vi "Read Tiff File (Bitmiracle libtiff.net).vi"(8 "error in (no error)":errorcluster, 11 "Input path":path=path "C:/0_DLPGUI_V2/lowResTest.tif") -> (0 "error out":errorcluster, 2 "ImageData":T1, 3 "Grayscale (U16) Image Data":u16[][][](array[numeric]), 4 "number of frames":i32)   [LabVIEW 2022 SP3]
doc: "This SubVI is a modified version of the file Read Tiff File.vi that is included in the libtiff2.llb library. The libtiff2.llb was provided by Nico_MPI on the NI LabVIEW discussion forum at http://forums.ni.com/t5/LabVIEW/Labview-libtiff-implementation/td-p/929843/page/2.\n\nRead a multipage TIFF returning an array of images and the total number of frames. This VI closes the file after returning the images array."
uses:
  Classes/TopLevel/Typedefs/TiffImageData--Cluster.ctl
  <vilib>/LVH/i3 JSON/JSON Parsing/Get Object Parameter Files/Get Object Parameter - Object.vi
  <vilib>/LVH/i3 JSON/JSON Parsing/Get Array Value at Index Files/Get Array Value at Index - Array.vi
  C:/Nuget/BitMiracle.LibTiff.NET.2.4.649/lib/net40/BitMiracle.LibTiff.NET.dll
  Nuget/BitMiracle.LibTiff.NET.2.4.649/lib/net40/BitMiracle.LibTiff.NET.dll
  BitMiracle.LibTiff.NET.dll
  <vilib>/LVH/i3 JSON/i3-json.lvlib
panel:
  out "Numeric":i32
  out "ImageBufferMain":u8[][](array[numeric])
  out "ChannelTargetMaterials":string[](array[string])
  out "MaterialNames":string[](array[string])
  out "error out 2":errorcluster
  out "Subject":string
  out "0 6":T2(plugin-control)
  out "0 5":T2(plugin-control)
  out "0 4":T2(plugin-control)
  out "0 3":T2(plugin-control)
  out "0 2":T2(plugin-control)
  out "ScanLineSize":i32
  out "0":T2(plugin-control)
  out "element 2":i32
  out "unsigned 8bit integer":u8[][](array[numeric])
  out "buffer":u8[][](array[numeric])
  out "Array":u64[](array[numeric])
  out "element":i32
  out "NumberOfTiles":i32
  out "Number Bytes read 2":i32
  out "Number Bytes read":i32
  out "Grayscale (SGL) Image Data":sgl[][][](array[numeric])
  # "278x1271"
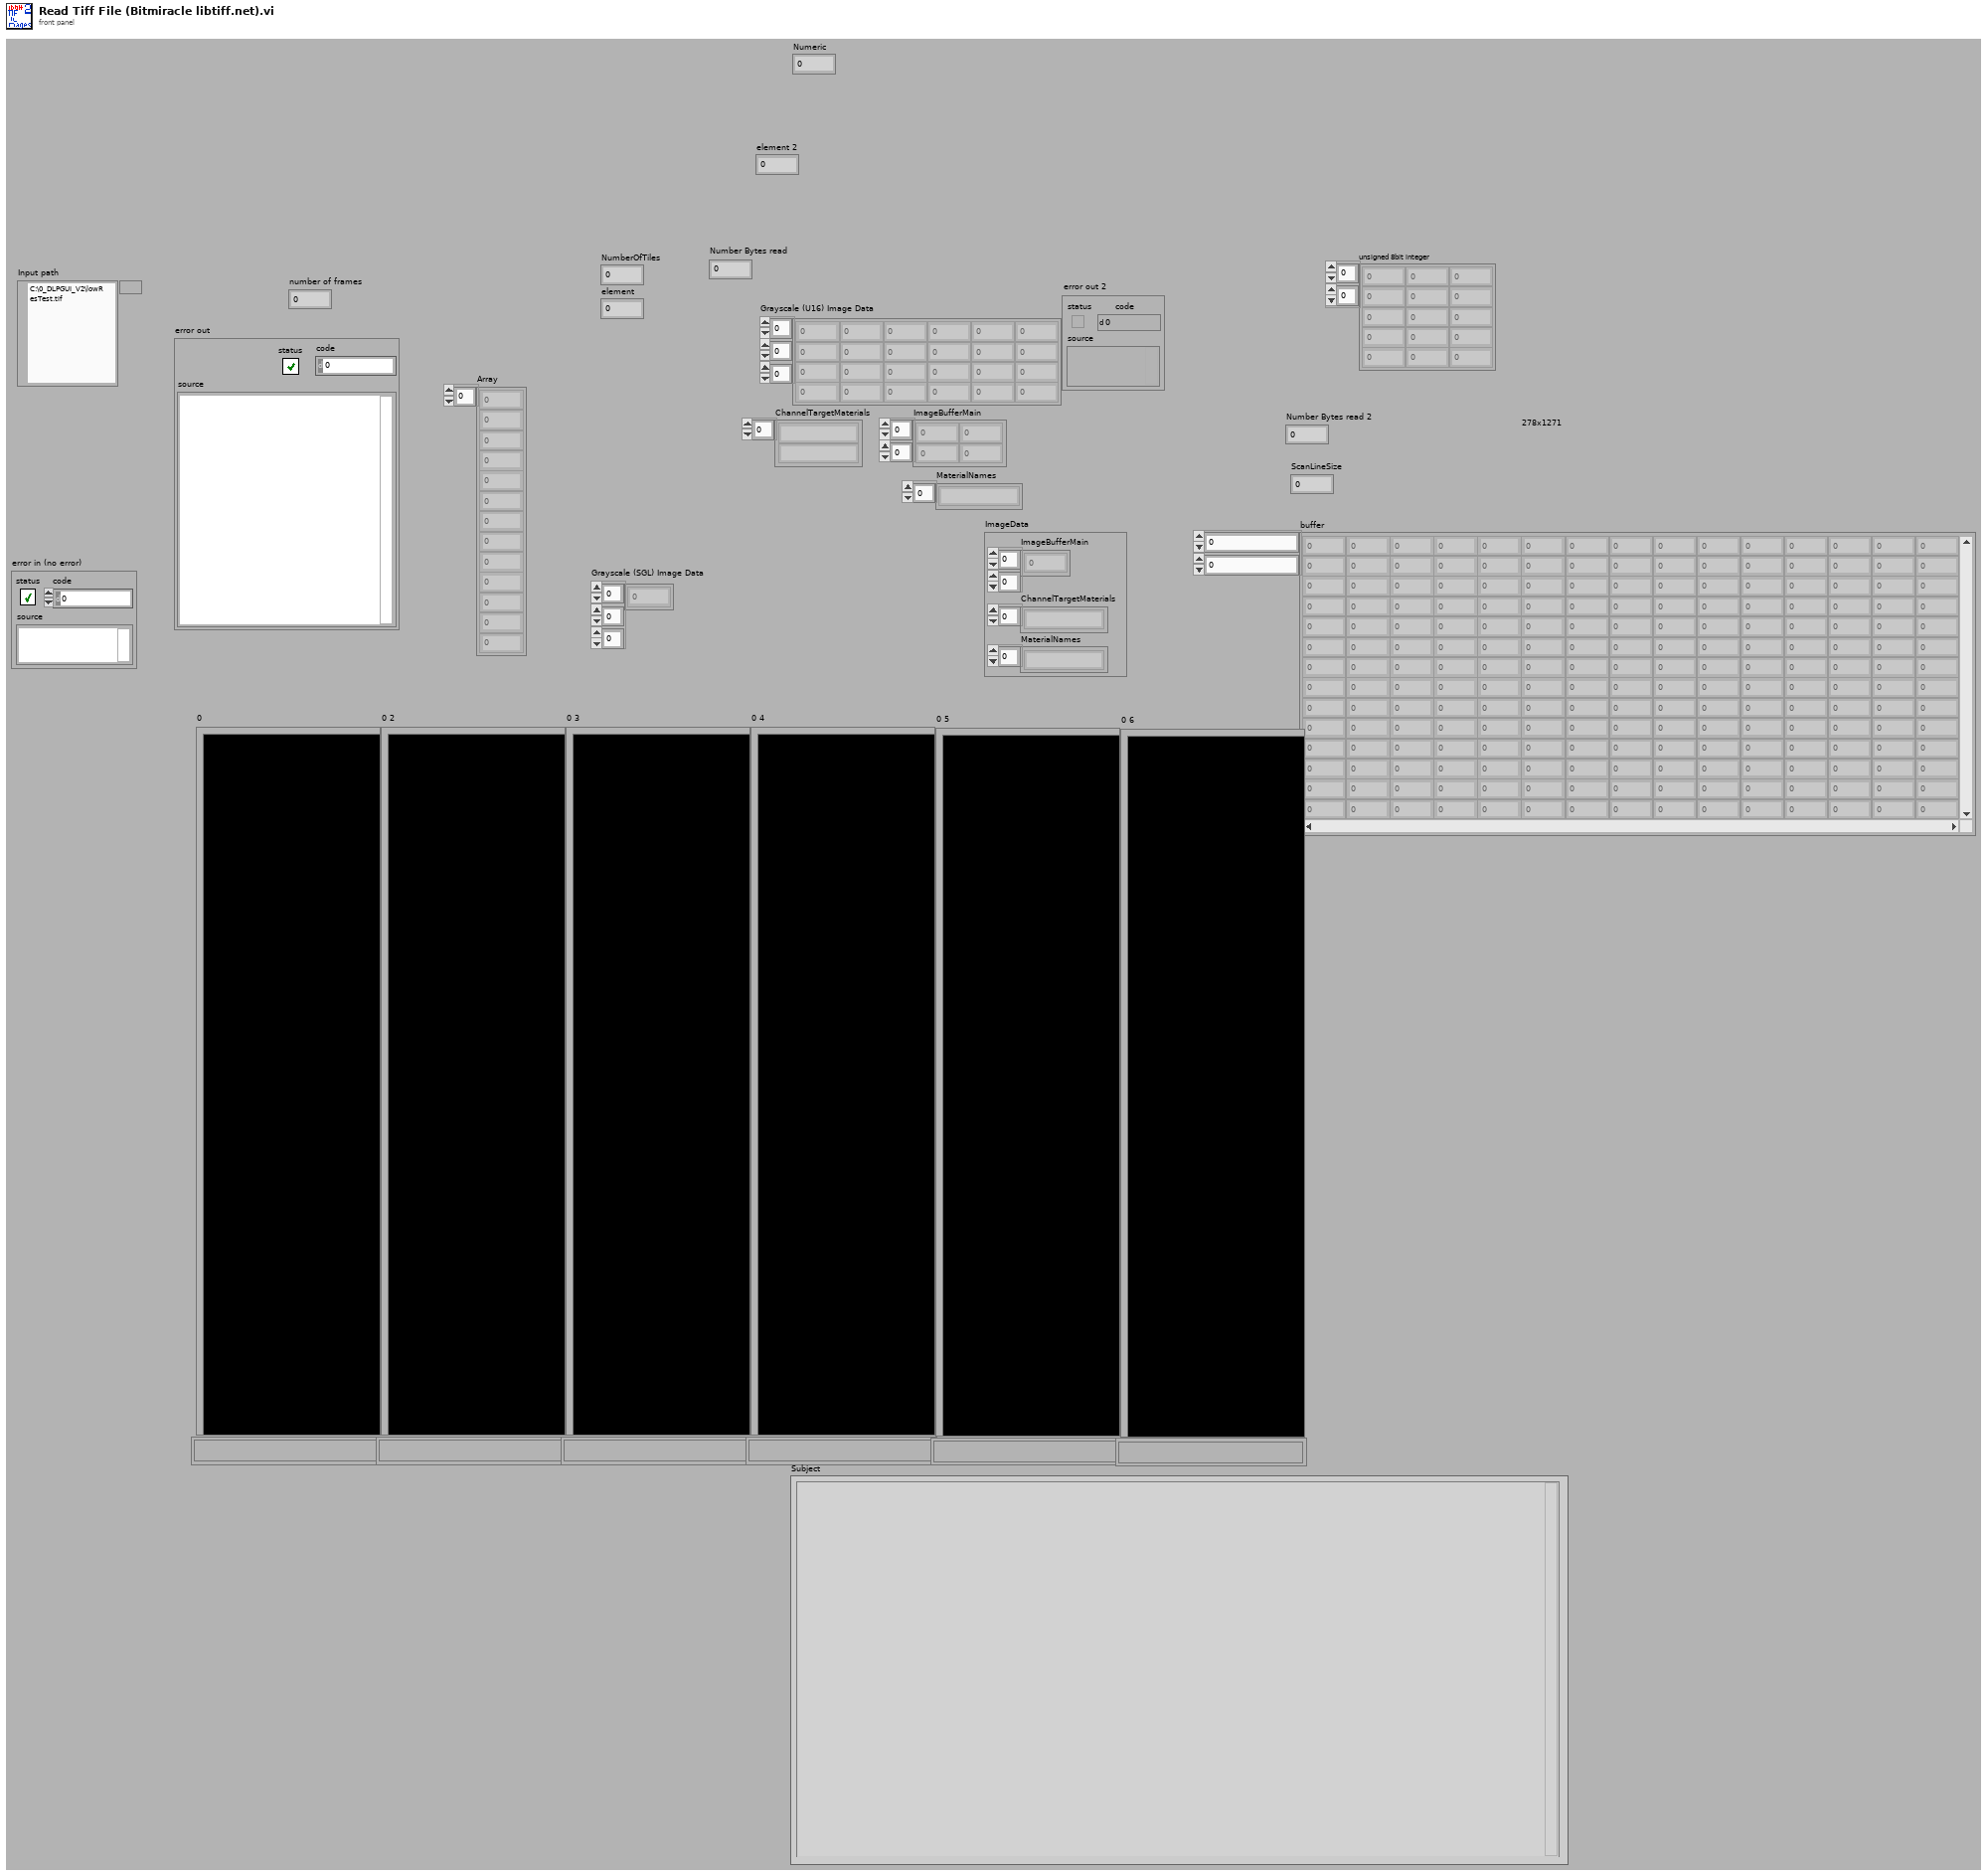
[diagram p1: front panel]
types:
  T1 = typedef "TiffImageData--Cluster.ctl" = cluster{"ImageBufferMain":u8[][], "ChannelTargetMaterials":string[], "MaterialNames":string[]}
  T2 = typedef "IMAQ Image.ctl" = refnum<image>
  T3 = typedef "Image Type" = u32
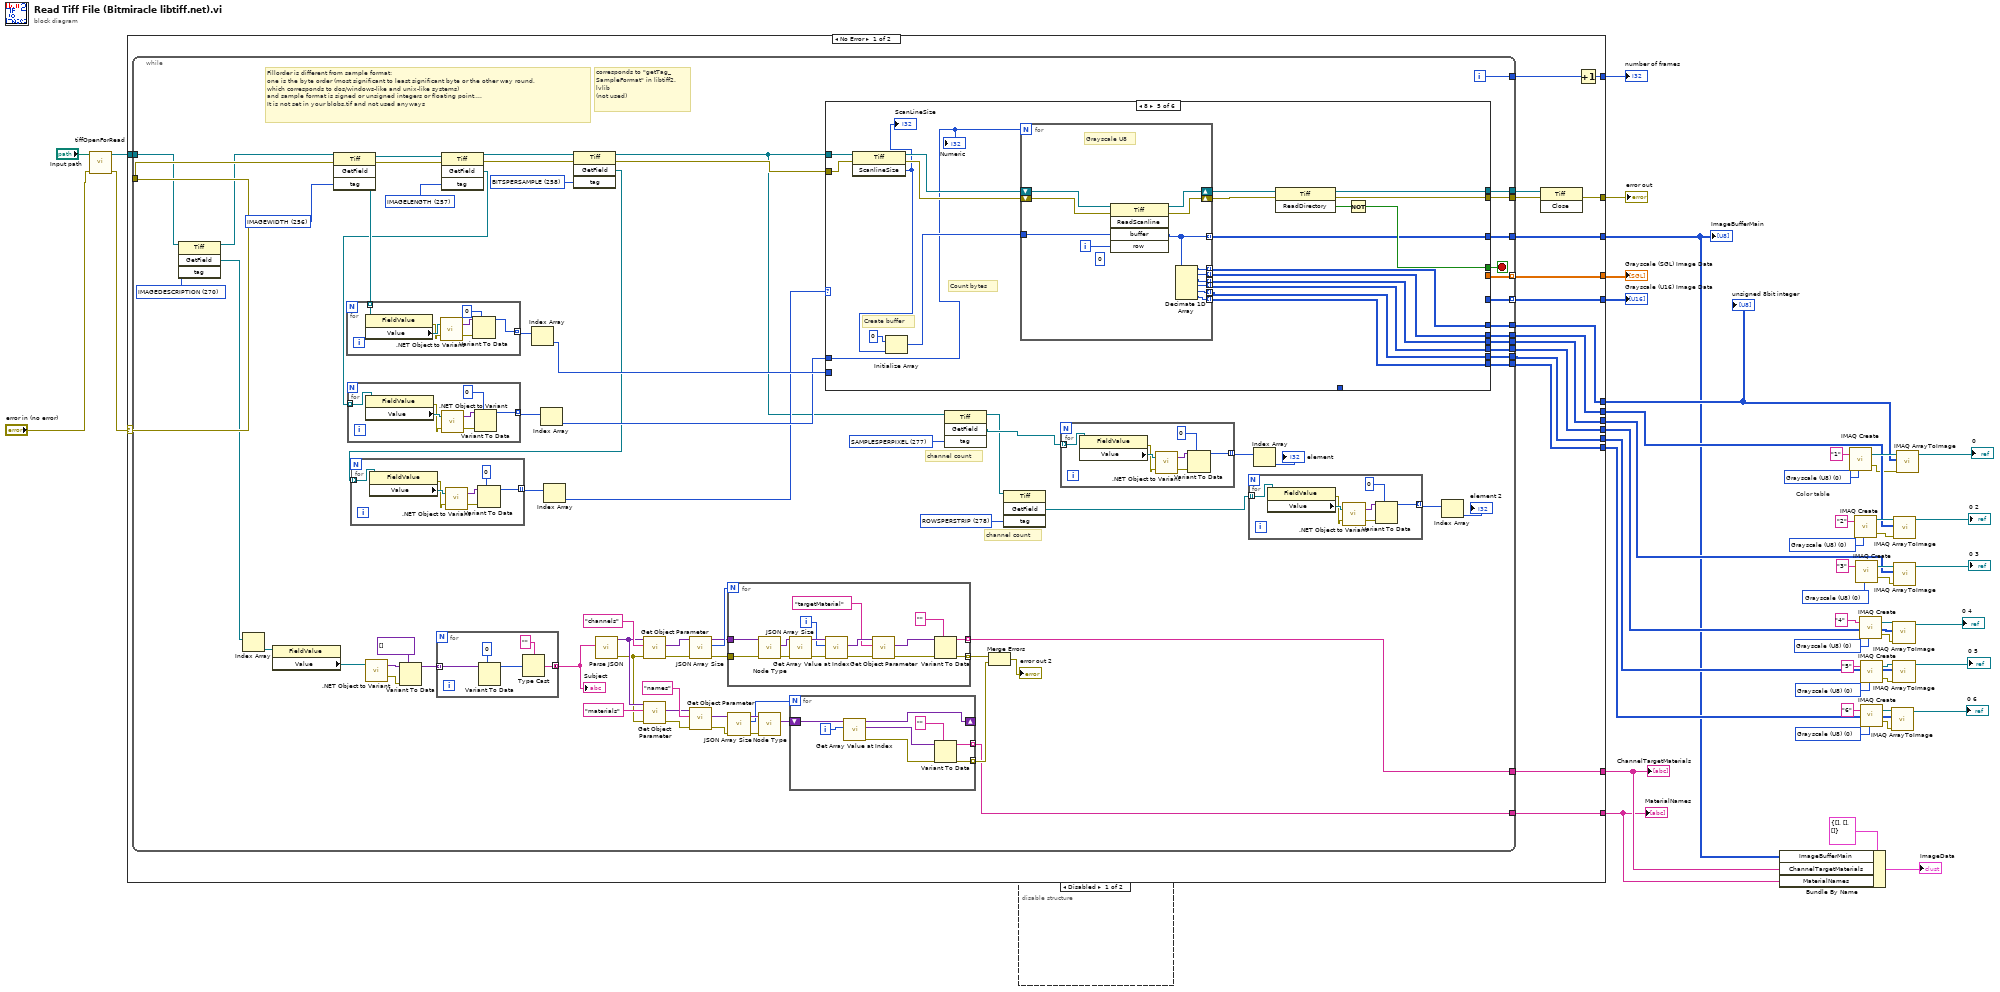
[diagram p0: block diagram]
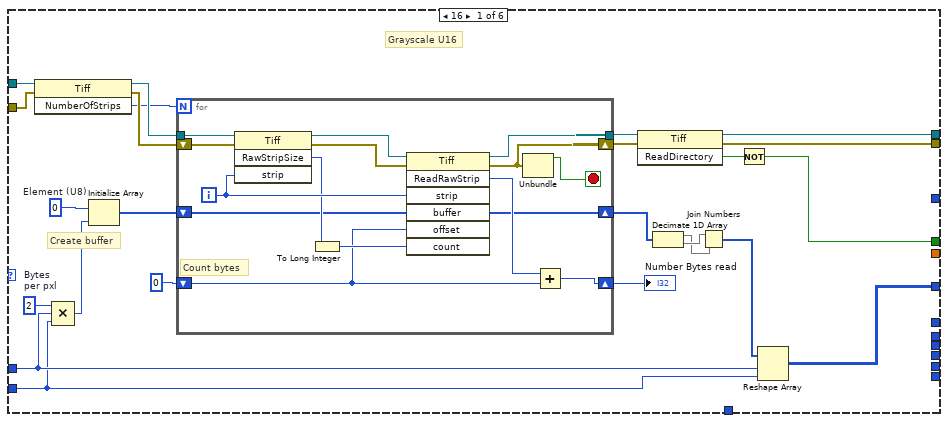
[diagram p3: hidden frame]
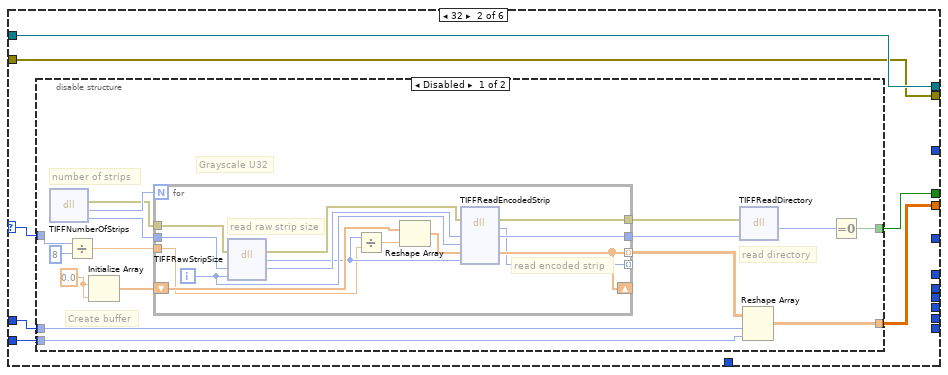
[diagram p4: hidden frame]
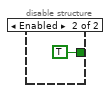
[diagram p5: hidden frame]
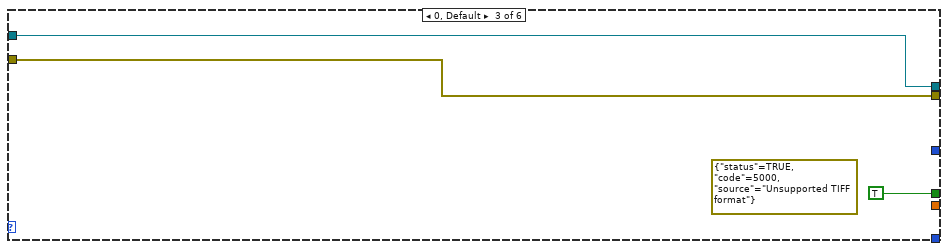
[diagram p6: hidden frame]
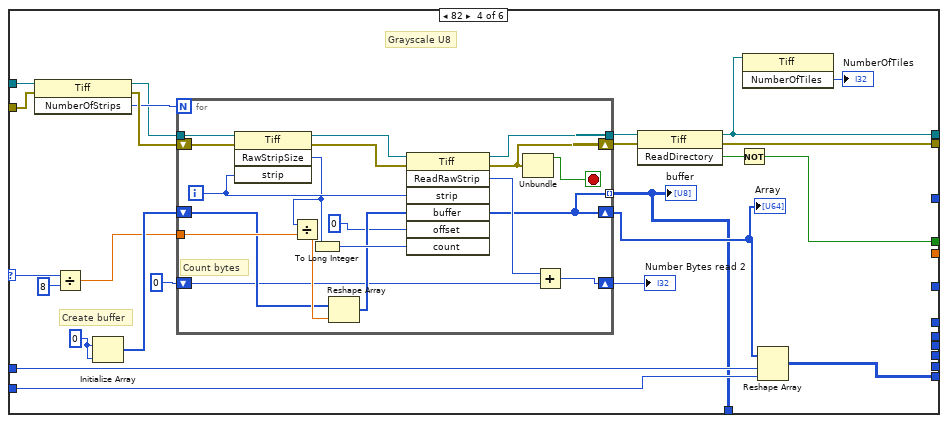
[diagram p7: hidden frame]
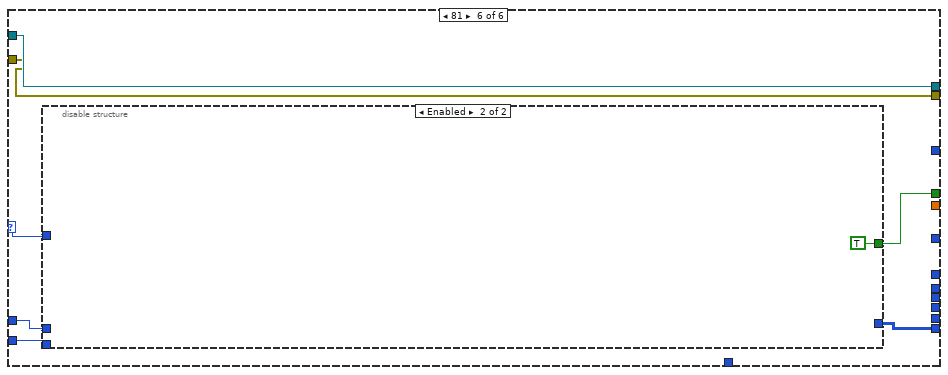
[diagram p8: hidden frame]
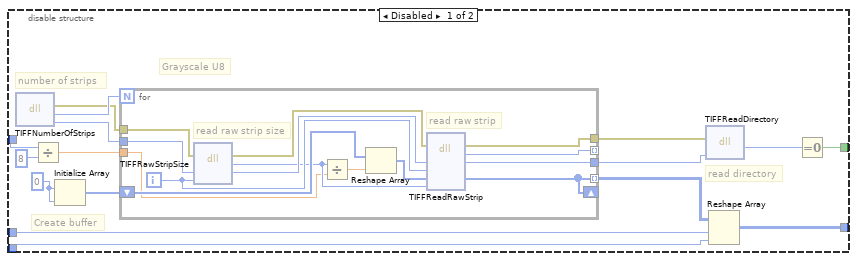
[diagram p9: hidden frame]
diagram:
  w27 = T3 0 items=["Grayscale (U8)", "Grayscale (I16)", "Grayscale (SGL)", "Complex (CSG)", "RGB (U32)", "HSL (U32)", "RGB (U64)", "Grayscale (U16)"] ("Image Type")
  w32 = T3 0 items=["Grayscale (U8)", "Grayscale (I16)", "Grayscale (SGL)", "Complex (CSG)", "RGB (U32)", "HSL (U32)", "RGB (U64)", "Grayscale (U16)"] ("Image Type")
  w29 = T3 0 items=["Grayscale (U8)", "Grayscale (I16)", "Grayscale (SGL)", "Complex (CSG)", "RGB (U32)", "HSL (U32)", "RGB (U64)", "Grayscale (U16)"] ("Image Type")
  w33 = T3 0 items=["Grayscale (U8)", "Grayscale (I16)", "Grayscale (SGL)", "Complex (CSG)", "RGB (U32)", "HSL (U32)", "RGB (U64)", "Grayscale (U16)"] ("Image Type")
  w36 = T3 0 items=["Grayscale (U8)", "Grayscale (I16)", "Grayscale (SGL)", "Complex (CSG)", "RGB (U32)", "HSL (U32)", "RGB (U64)", "Grayscale (U16)"] ("Image Type")
  w40 = T3 0 items=["Grayscale (U8)", "Grayscale (I16)", "Grayscale (SGL)", "Complex (CSG)", "RGB (U32)", "HSL (U32)", "RGB (U64)", "Grayscale (U16)"] ("Image Type")
  # "Color table"
  n1 = call "tiffOpenForRead.vi"("error in (no error)"="error in (no error)", "Path"="Input path") -> ("error out"=w42:errorcluster, "BitMiracle.LibTiff.Classic.Tiff"=w45:refnum<k24>)  [unwired: 8 in]
  n2 = case shown="No Error" w42 {
    selector: w42 -> [w67 w401]
    tunnel: [w65 _] -> w49
    tunnel: [w59 w401] -> w48
    tunnel: [w64 _] -> w47
    tunnel: [w63 _] -> w44
    tunnel: w45 -> [w62 _]
    tunnel: [w58 _] -> w37
    tunnel: [w57 _] -> w24
    tunnel: [w56 _] -> w9
    tunnel: [w55 _] -> w8
    tunnel: [w54 _] -> w7
    tunnel: [w53 _] -> w6
    tunnel: [w52 _] -> w3
    tunnel: [w51 _] -> w2
    tunnel: [w50 _] -> w1
    frame No Error {
      n3 = while {
        tunnel: [w141] -> w66
        tunnel: w67 -> [w102]
        tunnel: [w137] -> w63 mode=indexing
        tunnel: [w140] -> w64 mode=indexing
        tunnel: w62 -> [w101]
        tunnel: [w139] -> w61
        tunnel: [w138] -> w60
        tunnel: [w114] -> w53
        tunnel: [w108] -> w58
        tunnel: [w107] -> w57
        tunnel: [w106] -> w56
        tunnel: [w105] -> w55
        tunnel: [w104] -> w54
        tunnel: [w70] -> w52
        tunnel: [w69] -> w51
        tunnel: [w68] -> w50
        i -> [w141]
        stop <- w142 stop-if-true
        w103 = 270 items=["IGNORE"=0, "SUBFILETYPE"=254, "OSUBFILETYPE"=255, "IMAGEWIDTH"=256, "IMAGELENGTH"=257, "BITSPERSAMPLE"=258, "COMPRESSION"=259, "PHOTOMETRIC"=262, "THRESHHOLDING"=263, "CELLWIDTH"=264, "CELLLENGTH"=265, "FILLORDER"=266, "DOCUMENTNAME"=269, "IMAGEDESCRIPTION"=270, "MAKE"=271, "MODEL"=272, "STRIPOFFSETS"=273, "ORIENTATION"=274, "SAMPLESPERPIXEL"=277, "ROWSPERSTRIP"=278, "STRIPBYTECOUNTS"=279, "MINSAMPLEVALUE"=280, "MAXSAMPLEVALUE"=281, "XRESOLUTION"=282, "YRESOLUTION"=283, "PLANARCONFIG"=284, "PAGENAME"=285, "XPOSITION"=286, "YPOSITION"=287, "FREEOFFSETS"=288, "FREEBYTECOUNTS"=289, "GRAYRESPONSEUNIT"=290, "GRAYRESPONSECURVE"=291, "GROUP3OPTIONS, T4OPTIONS"=292, "GROUP4OPTIONS, T6OPTIONS"=293, "RESOLUTIONUNIT"=296, "PAGENUMBER"=297, "COLORRESPONSEUNIT"=300, "TRANSFERFUNCTION"=301, "SOFTWARE"=305, "DATETIME"=306, "ARTIST"=315, "HOSTCOMPUTER"=316, "PREDICTOR"=317, "WHITEPOINT"=318, "PRIMARYCHROMATICITIES"=319, "COLORMAP"=320, "HALFTONEHINTS"=321, "TILEWIDTH"=322, "TILELENGTH"=323, "TILEOFFSETS"=324, "TILEBYTECOUNTS"=325, "BADFAXLINES"=326, "CLEANFAXDATA"=327, "CONSECUTIVEBADFAXLINES"=328, "SUBIFD"=330, "INKSET"=332, "INKNAMES"=333, "NUMBEROFINKS"=334, "DOTRANGE"=336, "TARGETPRINTER"=337, "EXTRASAMPLES"=338, "SAMPLEFORMAT"=339, "SMINSAMPLEVALUE"=340, "SMAXSAMPLEVALUE"=341, "CLIPPATH"=343, "XCLIPPATHUNITS"=344, "YCLIPPATHUNITS"=345, "INDEXED"=346, "JPEGTABLES"=347, "OPIPROXY"=351, "JPEGPROC"=512, "JPEGIFOFFSET"=513, "JPEGIFBYTECOUNT"=514, "JPEGRESTARTINTERVAL"=515, "JPEGLOSSLESSPREDICTORS"=517, "JPEGPOINTTRANSFORM"=518, "JPEGQTABLES"=519, "JPEGDCTABLES"=520, "JPEGACTABLES"=521, "YCBCRCOEFFICIENTS"=529, "YCBCRSUBSAMPLING"=530, "YCBCRPOSITIONING"=531, "REFERENCEBLACKWHITE"=532, "XMLPACKET"=700, "OPIIMAGEID"=32781, "REFPTS"=32953, "REGIONTACKPOINT"=32954, "REGIONWARPCORNERS"=32955, "REGIONAFFINE"=32956, "MATTEING"=32995, "DATATYPE"=32996, "IMAGEDEPTH"=32997, "TILEDEPTH"=32998, "PIXAR_IMAGEFULLWIDTH"=33300, "PIXAR_IMAGEFULLLENGTH"=33301, "PIXAR_TEXTUREFORMAT"=33302, "PIXAR_WRAPMODES"=33303, "PIXAR_FOVCOT"=33304, "PIXAR_MATRIX_WORLDTOSCREEN"=33305, "PIXAR_MATRIX_WORLDTOCAMERA"=33306, "WRITERSERIALNUMBER"=33405, "COPYRIGHT"=33432, "EXIF_EXPOSURETIME"=33434, "EXIF_FNUMBER"=33437, "GEOTIFF_MODELPIXELSCALETAG"=33550, "RICHTIFFIPTC"=33723, "GEOTIFF_MODELTIEPOINTTAG"=33922, "IT8SITE"=34016, "IT8COLORSEQUENCE"=34017, "IT8HEADER"=34018, "IT8RASTERPADDING"=34019, "IT8BITSPERRUNLENGTH"=34020, "IT8BITSPEREXTENDEDRUNLENGTH"=34021, "IT8COLORTABLE"=34022, "IT8IMAGECOLORINDICATOR"=34023, "IT8BKGCOLORINDICATOR"=34024, "IT8IMAGECOLORVALUE"=34025, "IT8BKGCOLORVALUE"=34026, "IT8PIXELINTENSITYRANGE"=34027, "IT8TRANSPARENCYINDICATOR"=34028, "IT8COLORCHARACTERIZATION"=34029, "IT8HCUSAGE"=34030, "IT8TRAPINDICATOR"=34031, "IT8CMYKEQUIVALENT"=34032, "FRAMECOUNT"=34232, "GEOTIFF_MODELTRANSFORMATIONTAG"=34264, "PHOTOSHOP"=34377, "EXIFIFD"=34665, "ICCPROFILE"=34675, "GEOTIFF_GEOKEYDIRECTORYTAG"=34735, "GEOTIFF_GEODOUBLEPARAMSTAG"=34736, "GEOTIFF_GEOASCIIPARAMSTAG"=34737, "JBIGOPTIONS"=34750, "EXIF_EXPOSUREPROGRAM"=34850, "EXIF_SPECTRALSENSITIVITY"=34852, "GPSIFD"=34853, "EXIF_ISOSPEEDRATINGS"=34855, "EXIF_OECF"=34856, "FAXRECVPARAMS"=34908, "FAXSUBADDRESS"=34909, "FAXRECVTIME"=34910, "FAXDCS"=34911, "FEDEX_EDR"=34929, "EXIF_EXIFVERSION"=36864, "EXIF_DATETIMEORIGINAL"=36867, "EXIF_DATETIMEDIGITIZED"=36868, "EXIF_COMPONENTSCONFIGURATION"=37121, "EXIF_COMPRESSEDBITSPERPIXEL"=37122, "EXIF_SHUTTERSPEEDVALUE"=37377, "EXIF_APERTUREVALUE"=37378, "EXIF_BRIGHTNESSVALUE"=37379, "EXIF_EXPOSUREBIASVALUE"=37380, "EXIF_MAXAPERTUREVALUE"=37381, "EXIF_SUBJECTDISTANCE"=37382, "EXIF_METERINGMODE"=37383, "EXIF_LIGHTSOURCE"=37384, "EXIF_FLASH"=37385, "EXIF_FOCALLENGTH"=37386, "EXIF_SUBJECTAREA"=37396, "STONITS"=37439, "EXIF_MAKERNOTE"=37500, "EXIF_USERCOMMENT"=37510, "EXIF_SUBSECTIME"=37520, "EXIF_SUBSECTIMEORIGINAL"=37521, "EXIF_SUBSECTIMEDIGITIZED"=37522, "EXIF_FLASHPIXVERSION"=40960, "EXIF_COLORSPACE"=40961, "EXIF_PIXELXDIMENSION"=40962, "EXIF_PIXELYDIMENSION"=40963, "EXIF_RELATEDSOUNDFILE"=40964, "INTEROPERABILITYIFD"=40965, "EXIF_FLASHENERGY"=41483, "EXIF_SPATIALFREQUENCYRESPONSE"=41484, "EXIF_FOCALPLANEXRESOLUTION"=41486, "EXIF_FOCALPLANEYRESOLUTION"=41487, "EXIF_FOCALPLANERESOLUTIONUNIT"=41488, "EXIF_SUBJECTLOCATION"=41492, "EXIF_EXPOSUREINDEX"=41493, "EXIF_SENSINGMETHOD"=41495, "EXIF_FILESOURCE"=41728, "EXIF_SCENETYPE"=41729, "EXIF_CFAPATTERN"=41730, "EXIF_CUSTOMRENDERED"=41985, "EXIF_EXPOSUREMODE"=41986, "EXIF_WHITEBALANCE"=41987, "EXIF_DIGITALZOOMRATIO"=41988, "EXIF_FOCALLENGTHIN35MMFILM"=41989, "EXIF_SCENECAPTURETYPE"=41990, "EXIF_GAINCONTROL"=41991, "EXIF_CONTRAST"=41992, "EXIF_SATURATION"=41993, "EXIF_SHARPNESS"=41994, "EXIF_DEVICESETTINGDESCRIPTION"=41995, "EXIF_SUBJECTDISTANCERANGE"=41996, "EXIF_IMAGEUNIQUEID"=42016, "DNGVERSION"=50706, "DNGBACKWARDVERSION"=50707, "UNIQUECAMERAMODEL"=50708, "LOCALIZEDCAMERAMODEL"=50709, "CFAPLANECOLOR"=50710, "CFALAYOUT"=50711, "LINEARIZATIONTABLE"=50712, "BLACKLEVELREPEATDIM"=50713, "BLACKLEVEL"=50714, "BLACKLEVELDELTAH"=50715, "BLACKLEVELDELTAV"=50716, "WHITELEVEL"=50717, "DEFAULTSCALE"=50718, "DEFAULTCROPORIGIN"=50719, "DEFAULTCROPSIZE"=50720, "COLORMATRIX1"=50721, "COLORMATRIX2"=50722, "CAMERACALIBRATION1"=50723, "CAMERACALIBRATION2"=50724, "REDUCTIONMATRIX1"=50725, "REDUCTIONMATRIX2"=50726, "ANALOGBALANCE"=50727, "ASSHOTNEUTRAL"=50728, "ASSHOTWHITEXY"=50729, "BASELINEEXPOSURE"=50730, "BASELINENOISE"=50731, "BASELINESHARPNESS"=50732, "BAYERGREENSPLIT"=50733, "LINEARRESPONSELIMIT"=50734, "CAMERASERIALNUMBER"=50735, "LENSINFO"=50736, "CHROMABLURRADIUS"=50737, "ANTIALIASSTRENGTH"=50738, "SHADOWSCALE"=50739, "DNGPRIVATEDATA"=50740, "MAKERNOTESAFETY"=50741, "CALIBRATIONILLUMINANT1"=50778, "CALIBRATIONILLUMINANT2"=50779, "BESTQUALITYSCALE"=50780, "RAWDATAUNIQUEID"=50781, "ORIGINALRAWFILENAME"=50827, "ORIGINALRAWFILEDATA"=50828, "ACTIVEAREA"=50829, "MASKEDAREAS"=50830, "ASSHOTICCPROFILE"=50831, "ASSHOTPREPROFILEMATRIX"=50832, "CURRENTICCPROFILE"=50833, "CURRENTPREPROFILEMATRIX"=50834, "DCSHUESHIFTVALUES"=65535, "FAXMODE"=65536, "JPEGQUALITY"=65537, "JPEGCOLORMODE"=65538, "JPEGTABLESMODE"=65539, "FAXFILLFUNC"=65540, "PIXARLOGDATAFMT"=65549, "DCSIMAGERTYPE"=65550, "DCSINTERPMODE"=65551, "DCSBALANCEARRAY"=65552, "DCSCORRECTMATRIX"=65553, "DCSGAMMA"=65554, "DCSTOESHOULDERPTS"=65555, "DCSCALIBRATIONFD"=65556, "ZIPQUALITY"=65557, "PIXARLOGQUALITY"=65558, "DCSCLIPRECTANGLE"=65559, "SGILOGDATAFMT"=65560, "SGILOGENCODE"=65561] ("tag")
        w113 = 278 items=["IGNORE"=0, "SUBFILETYPE"=254, "OSUBFILETYPE"=255, "IMAGEWIDTH"=256, "IMAGELENGTH"=257, "BITSPERSAMPLE"=258, "COMPRESSION"=259, "PHOTOMETRIC"=262, "THRESHHOLDING"=263, "CELLWIDTH"=264, "CELLLENGTH"=265, "FILLORDER"=266, "DOCUMENTNAME"=269, "IMAGEDESCRIPTION"=270, "MAKE"=271, "MODEL"=272, "STRIPOFFSETS"=273, "ORIENTATION"=274, "SAMPLESPERPIXEL"=277, "ROWSPERSTRIP"=278, "STRIPBYTECOUNTS"=279, "MINSAMPLEVALUE"=280, "MAXSAMPLEVALUE"=281, "XRESOLUTION"=282, "YRESOLUTION"=283, "PLANARCONFIG"=284, "PAGENAME"=285, "XPOSITION"=286, "YPOSITION"=287, "FREEOFFSETS"=288, "FREEBYTECOUNTS"=289, "GRAYRESPONSEUNIT"=290, "GRAYRESPONSECURVE"=291, "GROUP3OPTIONS, T4OPTIONS"=292, "GROUP4OPTIONS, T6OPTIONS"=293, "RESOLUTIONUNIT"=296, "PAGENUMBER"=297, "COLORRESPONSEUNIT"=300, "TRANSFERFUNCTION"=301, "SOFTWARE"=305, "DATETIME"=306, "ARTIST"=315, "HOSTCOMPUTER"=316, "PREDICTOR"=317, "WHITEPOINT"=318, "PRIMARYCHROMATICITIES"=319, "COLORMAP"=320, "HALFTONEHINTS"=321, "TILEWIDTH"=322, "TILELENGTH"=323, "TILEOFFSETS"=324, "TILEBYTECOUNTS"=325, "BADFAXLINES"=326, "CLEANFAXDATA"=327, "CONSECUTIVEBADFAXLINES"=328, "SUBIFD"=330, "INKSET"=332, "INKNAMES"=333, "NUMBEROFINKS"=334, "DOTRANGE"=336, "TARGETPRINTER"=337, "EXTRASAMPLES"=338, "SAMPLEFORMAT"=339, "SMINSAMPLEVALUE"=340, "SMAXSAMPLEVALUE"=341, "CLIPPATH"=343, "XCLIPPATHUNITS"=344, "YCLIPPATHUNITS"=345, "INDEXED"=346, "JPEGTABLES"=347, "OPIPROXY"=351, "JPEGPROC"=512, "JPEGIFOFFSET"=513, "JPEGIFBYTECOUNT"=514, "JPEGRESTARTINTERVAL"=515, "JPEGLOSSLESSPREDICTORS"=517, "JPEGPOINTTRANSFORM"=518, "JPEGQTABLES"=519, "JPEGDCTABLES"=520, "JPEGACTABLES"=521, "YCBCRCOEFFICIENTS"=529, "YCBCRSUBSAMPLING"=530, "YCBCRPOSITIONING"=531, "REFERENCEBLACKWHITE"=532, "XMLPACKET"=700, "OPIIMAGEID"=32781, "REFPTS"=32953, "REGIONTACKPOINT"=32954, "REGIONWARPCORNERS"=32955, "REGIONAFFINE"=32956, "MATTEING"=32995, "DATATYPE"=32996, "IMAGEDEPTH"=32997, "TILEDEPTH"=32998, "PIXAR_IMAGEFULLWIDTH"=33300, "PIXAR_IMAGEFULLLENGTH"=33301, "PIXAR_TEXTUREFORMAT"=33302, "PIXAR_WRAPMODES"=33303, "PIXAR_FOVCOT"=33304, "PIXAR_MATRIX_WORLDTOSCREEN"=33305, "PIXAR_MATRIX_WORLDTOCAMERA"=33306, "WRITERSERIALNUMBER"=33405, "COPYRIGHT"=33432, "EXIF_EXPOSURETIME"=33434, "EXIF_FNUMBER"=33437, "RICHTIFFIPTC"=33723, "IT8SITE"=34016, "IT8COLORSEQUENCE"=34017, "IT8HEADER"=34018, "IT8RASTERPADDING"=34019, "IT8BITSPERRUNLENGTH"=34020, "IT8BITSPEREXTENDEDRUNLENGTH"=34021, "IT8COLORTABLE"=34022, "IT8IMAGECOLORINDICATOR"=34023, "IT8BKGCOLORINDICATOR"=34024, "IT8IMAGECOLORVALUE"=34025, "IT8BKGCOLORVALUE"=34026, "IT8PIXELINTENSITYRANGE"=34027, "IT8TRANSPARENCYINDICATOR"=34028, "IT8COLORCHARACTERIZATION"=34029, "IT8HCUSAGE"=34030, "IT8TRAPINDICATOR"=34031, "IT8CMYKEQUIVALENT"=34032, "FRAMECOUNT"=34232, "PHOTOSHOP"=34377, "EXIFIFD"=34665, "ICCPROFILE"=34675, "JBIGOPTIONS"=34750, "EXIF_EXPOSUREPROGRAM"=34850, "EXIF_SPECTRALSENSITIVITY"=34852, "GPSIFD"=34853, "EXIF_ISOSPEEDRATINGS"=34855, "EXIF_OECF"=34856, "FAXRECVPARAMS"=34908, "FAXSUBADDRESS"=34909, "FAXRECVTIME"=34910, "FAXDCS"=34911, "FEDEX_EDR"=34929, "EXIF_EXIFVERSION"=36864, "EXIF_DATETIMEORIGINAL"=36867, "EXIF_DATETIMEDIGITIZED"=36868, "EXIF_COMPONENTSCONFIGURATION"=37121, "EXIF_COMPRESSEDBITSPERPIXEL"=37122, "EXIF_SHUTTERSPEEDVALUE"=37377, "EXIF_APERTUREVALUE"=37378, "EXIF_BRIGHTNESSVALUE"=37379, "EXIF_EXPOSUREBIASVALUE"=37380, "EXIF_MAXAPERTUREVALUE"=37381, "EXIF_SUBJECTDISTANCE"=37382, "EXIF_METERINGMODE"=37383, "EXIF_LIGHTSOURCE"=37384, "EXIF_FLASH"=37385, "EXIF_FOCALLENGTH"=37386, "EXIF_SUBJECTAREA"=37396, "STONITS"=37439, "EXIF_MAKERNOTE"=37500, "EXIF_USERCOMMENT"=37510, "EXIF_SUBSECTIME"=37520, "EXIF_SUBSECTIMEORIGINAL"=37521, "EXIF_SUBSECTIMEDIGITIZED"=37522, "EXIF_FLASHPIXVERSION"=40960, "EXIF_COLORSPACE"=40961, "EXIF_PIXELXDIMENSION"=40962, "EXIF_PIXELYDIMENSION"=40963, "EXIF_RELATEDSOUNDFILE"=40964, "INTEROPERABILITYIFD"=40965, "EXIF_FLASHENERGY"=41483, "EXIF_SPATIALFREQUENCYRESPONSE"=41484, "EXIF_FOCALPLANEXRESOLUTION"=41486, "EXIF_FOCALPLANEYRESOLUTION"=41487, "EXIF_FOCALPLANERESOLUTIONUNIT"=41488, "EXIF_SUBJECTLOCATION"=41492, "EXIF_EXPOSUREINDEX"=41493, "EXIF_SENSINGMETHOD"=41495, "EXIF_FILESOURCE"=41728, "EXIF_SCENETYPE"=41729, "EXIF_CFAPATTERN"=41730, "EXIF_CUSTOMRENDERED"=41985, "EXIF_EXPOSUREMODE"=41986, "EXIF_WHITEBALANCE"=41987, "EXIF_DIGITALZOOMRATIO"=41988, "EXIF_FOCALLENGTHIN35MMFILM"=41989, "EXIF_SCENECAPTURETYPE"=41990, "EXIF_GAINCONTROL"=41991, "EXIF_CONTRAST"=41992, "EXIF_SATURATION"=41993, "EXIF_SHARPNESS"=41994, "EXIF_DEVICESETTINGDESCRIPTION"=41995, "EXIF_SUBJECTDISTANCERANGE"=41996, "EXIF_IMAGEUNIQUEID"=42016, "DNGVERSION"=50706, "DNGBACKWARDVERSION"=50707, "UNIQUECAMERAMODEL"=50708, "LOCALIZEDCAMERAMODEL"=50709, "CFAPLANECOLOR"=50710, "CFALAYOUT"=50711, "LINEARIZATIONTABLE"=50712, "BLACKLEVELREPEATDIM"=50713, "BLACKLEVEL"=50714, "BLACKLEVELDELTAH"=50715, "BLACKLEVELDELTAV"=50716, "WHITELEVEL"=50717, "DEFAULTSCALE"=50718, "DEFAULTCROPORIGIN"=50719, "DEFAULTCROPSIZE"=50720, "COLORMATRIX1"=50721, "COLORMATRIX2"=50722, "CAMERACALIBRATION1"=50723, "CAMERACALIBRATION2"=50724, "REDUCTIONMATRIX1"=50725, "REDUCTIONMATRIX2"=50726, "ANALOGBALANCE"=50727, "ASSHOTNEUTRAL"=50728, "ASSHOTWHITEXY"=50729, "BASELINEEXPOSURE"=50730, "BASELINENOISE"=50731, "BASELINESHARPNESS"=50732, "BAYERGREENSPLIT"=50733, "LINEARRESPONSELIMIT"=50734, "CAMERASERIALNUMBER"=50735, "LENSINFO"=50736, "CHROMABLURRADIUS"=50737, "ANTIALIASSTRENGTH"=50738, "SHADOWSCALE"=50739, "DNGPRIVATEDATA"=50740, "MAKERNOTESAFETY"=50741, "CALIBRATIONILLUMINANT1"=50778, "CALIBRATIONILLUMINANT2"=50779, "BESTQUALITYSCALE"=50780, "RAWDATAUNIQUEID"=50781, "ORIGINALRAWFILENAME"=50827, "ORIGINALRAWFILEDATA"=50828, "ACTIVEAREA"=50829, "MASKEDAREAS"=50830, "ASSHOTICCPROFILE"=50831, "ASSHOTPREPROFILEMATRIX"=50832, "CURRENTICCPROFILE"=50833, "CURRENTPREPROFILEMATRIX"=50834, "DCSHUESHIFTVALUES"=65535, "FAXMODE"=65536, "JPEGQUALITY"=65537, "JPEGCOLORMODE"=65538, "JPEGTABLESMODE"=65539, "FAXFILLFUNC"=65540, "PIXARLOGDATAFMT"=65549, "DCSIMAGERTYPE"=65550, "DCSINTERPMODE"=65551, "DCSBALANCEARRAY"=65552, "DCSCORRECTMATRIX"=65553, "DCSGAMMA"=65554, "DCSTOESHOULDERPTS"=65555, "DCSCALIBRATIONFD"=65556, "ZIPQUALITY"=65557, "PIXARLOGQUALITY"=65558, "DCSCLIPRECTANGLE"=65559, "SGILOGDATAFMT"=65560, "SGILOGENCODE"=65561] ("tag")
        w119 = 277 items=["IGNORE"=0, "SUBFILETYPE"=254, "OSUBFILETYPE"=255, "IMAGEWIDTH"=256, "IMAGELENGTH"=257, "BITSPERSAMPLE"=258, "COMPRESSION"=259, "PHOTOMETRIC"=262, "THRESHHOLDING"=263, "CELLWIDTH"=264, "CELLLENGTH"=265, "FILLORDER"=266, "DOCUMENTNAME"=269, "IMAGEDESCRIPTION"=270, "MAKE"=271, "MODEL"=272, "STRIPOFFSETS"=273, "ORIENTATION"=274, "SAMPLESPERPIXEL"=277, "ROWSPERSTRIP"=278, "STRIPBYTECOUNTS"=279, "MINSAMPLEVALUE"=280, "MAXSAMPLEVALUE"=281, "XRESOLUTION"=282, "YRESOLUTION"=283, "PLANARCONFIG"=284, "PAGENAME"=285, "XPOSITION"=286, "YPOSITION"=287, "FREEOFFSETS"=288, "FREEBYTECOUNTS"=289, "GRAYRESPONSEUNIT"=290, "GRAYRESPONSECURVE"=291, "GROUP3OPTIONS, T4OPTIONS"=292, "GROUP4OPTIONS, T6OPTIONS"=293, "RESOLUTIONUNIT"=296, "PAGENUMBER"=297, "COLORRESPONSEUNIT"=300, "TRANSFERFUNCTION"=301, "SOFTWARE"=305, "DATETIME"=306, "ARTIST"=315, "HOSTCOMPUTER"=316, "PREDICTOR"=317, "WHITEPOINT"=318, "PRIMARYCHROMATICITIES"=319, "COLORMAP"=320, "HALFTONEHINTS"=321, "TILEWIDTH"=322, "TILELENGTH"=323, "TILEOFFSETS"=324, "TILEBYTECOUNTS"=325, "BADFAXLINES"=326, "CLEANFAXDATA"=327, "CONSECUTIVEBADFAXLINES"=328, "SUBIFD"=330, "INKSET"=332, "INKNAMES"=333, "NUMBEROFINKS"=334, "DOTRANGE"=336, "TARGETPRINTER"=337, "EXTRASAMPLES"=338, "SAMPLEFORMAT"=339, "SMINSAMPLEVALUE"=340, "SMAXSAMPLEVALUE"=341, "CLIPPATH"=343, "XCLIPPATHUNITS"=344, "YCLIPPATHUNITS"=345, "INDEXED"=346, "JPEGTABLES"=347, "OPIPROXY"=351, "JPEGPROC"=512, "JPEGIFOFFSET"=513, "JPEGIFBYTECOUNT"=514, "JPEGRESTARTINTERVAL"=515, "JPEGLOSSLESSPREDICTORS"=517, "JPEGPOINTTRANSFORM"=518, "JPEGQTABLES"=519, "JPEGDCTABLES"=520, "JPEGACTABLES"=521, "YCBCRCOEFFICIENTS"=529, "YCBCRSUBSAMPLING"=530, "YCBCRPOSITIONING"=531, "REFERENCEBLACKWHITE"=532, "XMLPACKET"=700, "OPIIMAGEID"=32781, "REFPTS"=32953, "REGIONTACKPOINT"=32954, "REGIONWARPCORNERS"=32955, "REGIONAFFINE"=32956, "MATTEING"=32995, "DATATYPE"=32996, "IMAGEDEPTH"=32997, "TILEDEPTH"=32998, "PIXAR_IMAGEFULLWIDTH"=33300, "PIXAR_IMAGEFULLLENGTH"=33301, "PIXAR_TEXTUREFORMAT"=33302, "PIXAR_WRAPMODES"=33303, "PIXAR_FOVCOT"=33304, "PIXAR_MATRIX_WORLDTOSCREEN"=33305, "PIXAR_MATRIX_WORLDTOCAMERA"=33306, "WRITERSERIALNUMBER"=33405, "COPYRIGHT"=33432, "EXIF_EXPOSURETIME"=33434, "EXIF_FNUMBER"=33437, "RICHTIFFIPTC"=33723, "IT8SITE"=34016, "IT8COLORSEQUENCE"=34017, "IT8HEADER"=34018, "IT8RASTERPADDING"=34019, "IT8BITSPERRUNLENGTH"=34020, "IT8BITSPEREXTENDEDRUNLENGTH"=34021, "IT8COLORTABLE"=34022, "IT8IMAGECOLORINDICATOR"=34023, "IT8BKGCOLORINDICATOR"=34024, "IT8IMAGECOLORVALUE"=34025, "IT8BKGCOLORVALUE"=34026, "IT8PIXELINTENSITYRANGE"=34027, "IT8TRANSPARENCYINDICATOR"=34028, "IT8COLORCHARACTERIZATION"=34029, "IT8HCUSAGE"=34030, "IT8TRAPINDICATOR"=34031, "IT8CMYKEQUIVALENT"=34032, "FRAMECOUNT"=34232, "PHOTOSHOP"=34377, "EXIFIFD"=34665, "ICCPROFILE"=34675, "JBIGOPTIONS"=34750, "EXIF_EXPOSUREPROGRAM"=34850, "EXIF_SPECTRALSENSITIVITY"=34852, "GPSIFD"=34853, "EXIF_ISOSPEEDRATINGS"=34855, "EXIF_OECF"=34856, "FAXRECVPARAMS"=34908, "FAXSUBADDRESS"=34909, "FAXRECVTIME"=34910, "FAXDCS"=34911, "FEDEX_EDR"=34929, "EXIF_EXIFVERSION"=36864, "EXIF_DATETIMEORIGINAL"=36867, "EXIF_DATETIMEDIGITIZED"=36868, "EXIF_COMPONENTSCONFIGURATION"=37121, "EXIF_COMPRESSEDBITSPERPIXEL"=37122, "EXIF_SHUTTERSPEEDVALUE"=37377, "EXIF_APERTUREVALUE"=37378, "EXIF_BRIGHTNESSVALUE"=37379, "EXIF_EXPOSUREBIASVALUE"=37380, "EXIF_MAXAPERTUREVALUE"=37381, "EXIF_SUBJECTDISTANCE"=37382, "EXIF_METERINGMODE"=37383, "EXIF_LIGHTSOURCE"=37384, "EXIF_FLASH"=37385, "EXIF_FOCALLENGTH"=37386, "EXIF_SUBJECTAREA"=37396, "STONITS"=37439, "EXIF_MAKERNOTE"=37500, "EXIF_USERCOMMENT"=37510, "EXIF_SUBSECTIME"=37520, "EXIF_SUBSECTIMEORIGINAL"=37521, "EXIF_SUBSECTIMEDIGITIZED"=37522, "EXIF_FLASHPIXVERSION"=40960, "EXIF_COLORSPACE"=40961, "EXIF_PIXELXDIMENSION"=40962, "EXIF_PIXELYDIMENSION"=40963, "EXIF_RELATEDSOUNDFILE"=40964, "INTEROPERABILITYIFD"=40965, "EXIF_FLASHENERGY"=41483, "EXIF_SPATIALFREQUENCYRESPONSE"=41484, "EXIF_FOCALPLANEXRESOLUTION"=41486, "EXIF_FOCALPLANEYRESOLUTION"=41487, "EXIF_FOCALPLANERESOLUTIONUNIT"=41488, "EXIF_SUBJECTLOCATION"=41492, "EXIF_EXPOSUREINDEX"=41493, "EXIF_SENSINGMETHOD"=41495, "EXIF_FILESOURCE"=41728, "EXIF_SCENETYPE"=41729, "EXIF_CFAPATTERN"=41730, "EXIF_CUSTOMRENDERED"=41985, "EXIF_EXPOSUREMODE"=41986, "EXIF_WHITEBALANCE"=41987, "EXIF_DIGITALZOOMRATIO"=41988, "EXIF_FOCALLENGTHIN35MMFILM"=41989, "EXIF_SCENECAPTURETYPE"=41990, "EXIF_GAINCONTROL"=41991, "EXIF_CONTRAST"=41992, "EXIF_SATURATION"=41993, "EXIF_SHARPNESS"=41994, "EXIF_DEVICESETTINGDESCRIPTION"=41995, "EXIF_SUBJECTDISTANCERANGE"=41996, "EXIF_IMAGEUNIQUEID"=42016, "DNGVERSION"=50706, "DNGBACKWARDVERSION"=50707, "UNIQUECAMERAMODEL"=50708, "LOCALIZEDCAMERAMODEL"=50709, "CFAPLANECOLOR"=50710, "CFALAYOUT"=50711, "LINEARIZATIONTABLE"=50712, "BLACKLEVELREPEATDIM"=50713, "BLACKLEVEL"=50714, "BLACKLEVELDELTAH"=50715, "BLACKLEVELDELTAV"=50716, "WHITELEVEL"=50717, "DEFAULTSCALE"=50718, "DEFAULTCROPORIGIN"=50719, "DEFAULTCROPSIZE"=50720, "COLORMATRIX1"=50721, "COLORMATRIX2"=50722, "CAMERACALIBRATION1"=50723, "CAMERACALIBRATION2"=50724, "REDUCTIONMATRIX1"=50725, "REDUCTIONMATRIX2"=50726, "ANALOGBALANCE"=50727, "ASSHOTNEUTRAL"=50728, "ASSHOTWHITEXY"=50729, "BASELINEEXPOSURE"=50730, "BASELINENOISE"=50731, "BASELINESHARPNESS"=50732, "BAYERGREENSPLIT"=50733, "LINEARRESPONSELIMIT"=50734, "CAMERASERIALNUMBER"=50735, "LENSINFO"=50736, "CHROMABLURRADIUS"=50737, "ANTIALIASSTRENGTH"=50738, "SHADOWSCALE"=50739, "DNGPRIVATEDATA"=50740, "MAKERNOTESAFETY"=50741, "CALIBRATIONILLUMINANT1"=50778, "CALIBRATIONILLUMINANT2"=50779, "BESTQUALITYSCALE"=50780, "RAWDATAUNIQUEID"=50781, "ORIGINALRAWFILENAME"=50827, "ORIGINALRAWFILEDATA"=50828, "ACTIVEAREA"=50829, "MASKEDAREAS"=50830, "ASSHOTICCPROFILE"=50831, "ASSHOTPREPROFILEMATRIX"=50832, "CURRENTICCPROFILE"=50833, "CURRENTPREPROFILEMATRIX"=50834, "DCSHUESHIFTVALUES"=65535, "FAXMODE"=65536, "JPEGQUALITY"=65537, "JPEGCOLORMODE"=65538, "JPEGTABLESMODE"=65539, "FAXFILLFUNC"=65540, "PIXARLOGDATAFMT"=65549, "DCSIMAGERTYPE"=65550, "DCSINTERPMODE"=65551, "DCSBALANCEARRAY"=65552, "DCSCORRECTMATRIX"=65553, "DCSGAMMA"=65554, "DCSTOESHOULDERPTS"=65555, "DCSCALIBRATIONFD"=65556, "ZIPQUALITY"=65557, "PIXARLOGQUALITY"=65558, "DCSCLIPRECTANGLE"=65559, "SGILOGDATAFMT"=65560, "SGILOGENCODE"=65561] ("tag")
        w130 = 258 items=["IGNORE"=0, "SUBFILETYPE"=254, "OSUBFILETYPE"=255, "IMAGEWIDTH"=256, "IMAGELENGTH"=257, "BITSPERSAMPLE"=258, "COMPRESSION"=259, "PHOTOMETRIC"=262, "THRESHHOLDING"=263, "CELLWIDTH"=264, "CELLLENGTH"=265, "FILLORDER"=266, "DOCUMENTNAME"=269, "IMAGEDESCRIPTION"=270, "MAKE"=271, "MODEL"=272, "STRIPOFFSETS"=273, "ORIENTATION"=274, "SAMPLESPERPIXEL"=277, "ROWSPERSTRIP"=278, "STRIPBYTECOUNTS"=279, "MINSAMPLEVALUE"=280, "MAXSAMPLEVALUE"=281, "XRESOLUTION"=282, "YRESOLUTION"=283, "PLANARCONFIG"=284, "PAGENAME"=285, "XPOSITION"=286, "YPOSITION"=287, "FREEOFFSETS"=288, "FREEBYTECOUNTS"=289, "GRAYRESPONSEUNIT"=290, "GRAYRESPONSECURVE"=291, "GROUP3OPTIONS, T4OPTIONS"=292, "GROUP4OPTIONS, T6OPTIONS"=293, "RESOLUTIONUNIT"=296, "PAGENUMBER"=297, "COLORRESPONSEUNIT"=300, "TRANSFERFUNCTION"=301, "SOFTWARE"=305, "DATETIME"=306, "ARTIST"=315, "HOSTCOMPUTER"=316, "PREDICTOR"=317, "WHITEPOINT"=318, "PRIMARYCHROMATICITIES"=319, "COLORMAP"=320, "HALFTONEHINTS"=321, "TILEWIDTH"=322, "TILELENGTH"=323, "TILEOFFSETS"=324, "TILEBYTECOUNTS"=325, "BADFAXLINES"=326, "CLEANFAXDATA"=327, "CONSECUTIVEBADFAXLINES"=328, "SUBIFD"=330, "INKSET"=332, "INKNAMES"=333, "NUMBEROFINKS"=334, "DOTRANGE"=336, "TARGETPRINTER"=337, "EXTRASAMPLES"=338, "SAMPLEFORMAT"=339, "SMINSAMPLEVALUE"=340, "SMAXSAMPLEVALUE"=341, "CLIPPATH"=343, "XCLIPPATHUNITS"=344, "YCLIPPATHUNITS"=345, "INDEXED"=346, "JPEGTABLES"=347, "OPIPROXY"=351, "JPEGPROC"=512, "JPEGIFOFFSET"=513, "JPEGIFBYTECOUNT"=514, "JPEGRESTARTINTERVAL"=515, "JPEGLOSSLESSPREDICTORS"=517, "JPEGPOINTTRANSFORM"=518, "JPEGQTABLES"=519, "JPEGDCTABLES"=520, "JPEGACTABLES"=521, "YCBCRCOEFFICIENTS"=529, "YCBCRSUBSAMPLING"=530, "YCBCRPOSITIONING"=531, "REFERENCEBLACKWHITE"=532, "XMLPACKET"=700, "OPIIMAGEID"=32781, "REFPTS"=32953, "REGIONTACKPOINT"=32954, "REGIONWARPCORNERS"=32955, "REGIONAFFINE"=32956, "MATTEING"=32995, "DATATYPE"=32996, "IMAGEDEPTH"=32997, "TILEDEPTH"=32998, "PIXAR_IMAGEFULLWIDTH"=33300, "PIXAR_IMAGEFULLLENGTH"=33301, "PIXAR_TEXTUREFORMAT"=33302, "PIXAR_WRAPMODES"=33303, "PIXAR_FOVCOT"=33304, "PIXAR_MATRIX_WORLDTOSCREEN"=33305, "PIXAR_MATRIX_WORLDTOCAMERA"=33306, "WRITERSERIALNUMBER"=33405, "COPYRIGHT"=33432, "EXIF_EXPOSURETIME"=33434, "EXIF_FNUMBER"=33437, "RICHTIFFIPTC"=33723, "IT8SITE"=34016, "IT8COLORSEQUENCE"=34017, "IT8HEADER"=34018, "IT8RASTERPADDING"=34019, "IT8BITSPERRUNLENGTH"=34020, "IT8BITSPEREXTENDEDRUNLENGTH"=34021, "IT8COLORTABLE"=34022, "IT8IMAGECOLORINDICATOR"=34023, "IT8BKGCOLORINDICATOR"=34024, "IT8IMAGECOLORVALUE"=34025, "IT8BKGCOLORVALUE"=34026, "IT8PIXELINTENSITYRANGE"=34027, "IT8TRANSPARENCYINDICATOR"=34028, "IT8COLORCHARACTERIZATION"=34029, "IT8HCUSAGE"=34030, "IT8TRAPINDICATOR"=34031, "IT8CMYKEQUIVALENT"=34032, "FRAMECOUNT"=34232, "PHOTOSHOP"=34377, "EXIFIFD"=34665, "ICCPROFILE"=34675, "JBIGOPTIONS"=34750, "EXIF_EXPOSUREPROGRAM"=34850, "EXIF_SPECTRALSENSITIVITY"=34852, "GPSIFD"=34853, "EXIF_ISOSPEEDRATINGS"=34855, "EXIF_OECF"=34856, "FAXRECVPARAMS"=34908, "FAXSUBADDRESS"=34909, "FAXRECVTIME"=34910, "FAXDCS"=34911, "FEDEX_EDR"=34929, "EXIF_EXIFVERSION"=36864, "EXIF_DATETIMEORIGINAL"=36867, "EXIF_DATETIMEDIGITIZED"=36868, "EXIF_COMPONENTSCONFIGURATION"=37121, "EXIF_COMPRESSEDBITSPERPIXEL"=37122, "EXIF_SHUTTERSPEEDVALUE"=37377, "EXIF_APERTUREVALUE"=37378, "EXIF_BRIGHTNESSVALUE"=37379, "EXIF_EXPOSUREBIASVALUE"=37380, "EXIF_MAXAPERTUREVALUE"=37381, "EXIF_SUBJECTDISTANCE"=37382, "EXIF_METERINGMODE"=37383, "EXIF_LIGHTSOURCE"=37384, "EXIF_FLASH"=37385, "EXIF_FOCALLENGTH"=37386, "EXIF_SUBJECTAREA"=37396, "STONITS"=37439, "EXIF_MAKERNOTE"=37500, "EXIF_USERCOMMENT"=37510, "EXIF_SUBSECTIME"=37520, "EXIF_SUBSECTIMEORIGINAL"=37521, "EXIF_SUBSECTIMEDIGITIZED"=37522, "EXIF_FLASHPIXVERSION"=40960, "EXIF_COLORSPACE"=40961, "EXIF_PIXELXDIMENSION"=40962, "EXIF_PIXELYDIMENSION"=40963, "EXIF_RELATEDSOUNDFILE"=40964, "INTEROPERABILITYIFD"=40965, "EXIF_FLASHENERGY"=41483, "EXIF_SPATIALFREQUENCYRESPONSE"=41484, "EXIF_FOCALPLANEXRESOLUTION"=41486, "EXIF_FOCALPLANEYRESOLUTION"=41487, "EXIF_FOCALPLANERESOLUTIONUNIT"=41488, "EXIF_SUBJECTLOCATION"=41492, "EXIF_EXPOSUREINDEX"=41493, "EXIF_SENSINGMETHOD"=41495, "EXIF_FILESOURCE"=41728, "EXIF_SCENETYPE"=41729, "EXIF_CFAPATTERN"=41730, "EXIF_CUSTOMRENDERED"=41985, "EXIF_EXPOSUREMODE"=41986, "EXIF_WHITEBALANCE"=41987, "EXIF_DIGITALZOOMRATIO"=41988, "EXIF_FOCALLENGTHIN35MMFILM"=41989, "EXIF_SCENECAPTURETYPE"=41990, "EXIF_GAINCONTROL"=41991, "EXIF_CONTRAST"=41992, "EXIF_SATURATION"=41993, "EXIF_SHARPNESS"=41994, "EXIF_DEVICESETTINGDESCRIPTION"=41995, "EXIF_SUBJECTDISTANCERANGE"=41996, "EXIF_IMAGEUNIQUEID"=42016, "DNGVERSION"=50706, "DNGBACKWARDVERSION"=50707, "UNIQUECAMERAMODEL"=50708, "LOCALIZEDCAMERAMODEL"=50709, "CFAPLANECOLOR"=50710, "CFALAYOUT"=50711, "LINEARIZATIONTABLE"=50712, "BLACKLEVELREPEATDIM"=50713, "BLACKLEVEL"=50714, "BLACKLEVELDELTAH"=50715, "BLACKLEVELDELTAV"=50716, "WHITELEVEL"=50717, "DEFAULTSCALE"=50718, "DEFAULTCROPORIGIN"=50719, "DEFAULTCROPSIZE"=50720, "COLORMATRIX1"=50721, "COLORMATRIX2"=50722, "CAMERACALIBRATION1"=50723, "CAMERACALIBRATION2"=50724, "REDUCTIONMATRIX1"=50725, "REDUCTIONMATRIX2"=50726, "ANALOGBALANCE"=50727, "ASSHOTNEUTRAL"=50728, "ASSHOTWHITEXY"=50729, "BASELINEEXPOSURE"=50730, "BASELINENOISE"=50731, "BASELINESHARPNESS"=50732, "BAYERGREENSPLIT"=50733, "LINEARRESPONSELIMIT"=50734, "CAMERASERIALNUMBER"=50735, "LENSINFO"=50736, "CHROMABLURRADIUS"=50737, "ANTIALIASSTRENGTH"=50738, "SHADOWSCALE"=50739, "DNGPRIVATEDATA"=50740, "MAKERNOTESAFETY"=50741, "CALIBRATIONILLUMINANT1"=50778, "CALIBRATIONILLUMINANT2"=50779, "BESTQUALITYSCALE"=50780, "RAWDATAUNIQUEID"=50781, "ORIGINALRAWFILENAME"=50827, "ORIGINALRAWFILEDATA"=50828, "ACTIVEAREA"=50829, "MASKEDAREAS"=50830, "ASSHOTICCPROFILE"=50831, "ASSHOTPREPROFILEMATRIX"=50832, "CURRENTICCPROFILE"=50833, "CURRENTPREPROFILEMATRIX"=50834, "DCSHUESHIFTVALUES"=65535, "FAXMODE"=65536, "JPEGQUALITY"=65537, "JPEGCOLORMODE"=65538, "JPEGTABLESMODE"=65539, "FAXFILLFUNC"=65540, "PIXARLOGDATAFMT"=65549, "DCSIMAGERTYPE"=65550, "DCSINTERPMODE"=65551, "DCSBALANCEARRAY"=65552, "DCSCORRECTMATRIX"=65553, "DCSGAMMA"=65554, "DCSTOESHOULDERPTS"=65555, "DCSCALIBRATIONFD"=65556, "ZIPQUALITY"=65557, "PIXARLOGQUALITY"=65558, "DCSCLIPRECTANGLE"=65559, "SGILOGDATAFMT"=65560, "SGILOGENCODE"=65561] ("tag")
        w135 = 257 items=["IGNORE"=0, "SUBFILETYPE"=254, "OSUBFILETYPE"=255, "IMAGEWIDTH"=256, "IMAGELENGTH"=257, "BITSPERSAMPLE"=258, "COMPRESSION"=259, "PHOTOMETRIC"=262, "THRESHHOLDING"=263, "CELLWIDTH"=264, "CELLLENGTH"=265, "FILLORDER"=266, "DOCUMENTNAME"=269, "IMAGEDESCRIPTION"=270, "MAKE"=271, "MODEL"=272, "STRIPOFFSETS"=273, "ORIENTATION"=274, "SAMPLESPERPIXEL"=277, "ROWSPERSTRIP"=278, "STRIPBYTECOUNTS"=279, "MINSAMPLEVALUE"=280, "MAXSAMPLEVALUE"=281, "XRESOLUTION"=282, "YRESOLUTION"=283, "PLANARCONFIG"=284, "PAGENAME"=285, "XPOSITION"=286, "YPOSITION"=287, "FREEOFFSETS"=288, "FREEBYTECOUNTS"=289, "GRAYRESPONSEUNIT"=290, "GRAYRESPONSECURVE"=291, "GROUP3OPTIONS, T4OPTIONS"=292, "GROUP4OPTIONS, T6OPTIONS"=293, "RESOLUTIONUNIT"=296, "PAGENUMBER"=297, "COLORRESPONSEUNIT"=300, "TRANSFERFUNCTION"=301, "SOFTWARE"=305, "DATETIME"=306, "ARTIST"=315, "HOSTCOMPUTER"=316, "PREDICTOR"=317, "WHITEPOINT"=318, "PRIMARYCHROMATICITIES"=319, "COLORMAP"=320, "HALFTONEHINTS"=321, "TILEWIDTH"=322, "TILELENGTH"=323, "TILEOFFSETS"=324, "TILEBYTECOUNTS"=325, "BADFAXLINES"=326, "CLEANFAXDATA"=327, "CONSECUTIVEBADFAXLINES"=328, "SUBIFD"=330, "INKSET"=332, "INKNAMES"=333, "NUMBEROFINKS"=334, "DOTRANGE"=336, "TARGETPRINTER"=337, "EXTRASAMPLES"=338, "SAMPLEFORMAT"=339, "SMINSAMPLEVALUE"=340, "SMAXSAMPLEVALUE"=341, "CLIPPATH"=343, "XCLIPPATHUNITS"=344, "YCLIPPATHUNITS"=345, "INDEXED"=346, "JPEGTABLES"=347, "OPIPROXY"=351, "JPEGPROC"=512, "JPEGIFOFFSET"=513, "JPEGIFBYTECOUNT"=514, "JPEGRESTARTINTERVAL"=515, "JPEGLOSSLESSPREDICTORS"=517, "JPEGPOINTTRANSFORM"=518, "JPEGQTABLES"=519, "JPEGDCTABLES"=520, "JPEGACTABLES"=521, "YCBCRCOEFFICIENTS"=529, "YCBCRSUBSAMPLING"=530, "YCBCRPOSITIONING"=531, "REFERENCEBLACKWHITE"=532, "XMLPACKET"=700, "OPIIMAGEID"=32781, "REFPTS"=32953, "REGIONTACKPOINT"=32954, "REGIONWARPCORNERS"=32955, "REGIONAFFINE"=32956, "MATTEING"=32995, "DATATYPE"=32996, "IMAGEDEPTH"=32997, "TILEDEPTH"=32998, "PIXAR_IMAGEFULLWIDTH"=33300, "PIXAR_IMAGEFULLLENGTH"=33301, "PIXAR_TEXTUREFORMAT"=33302, "PIXAR_WRAPMODES"=33303, "PIXAR_FOVCOT"=33304, "PIXAR_MATRIX_WORLDTOSCREEN"=33305, "PIXAR_MATRIX_WORLDTOCAMERA"=33306, "WRITERSERIALNUMBER"=33405, "COPYRIGHT"=33432, "EXIF_EXPOSURETIME"=33434, "EXIF_FNUMBER"=33437, "RICHTIFFIPTC"=33723, "IT8SITE"=34016, "IT8COLORSEQUENCE"=34017, "IT8HEADER"=34018, "IT8RASTERPADDING"=34019, "IT8BITSPERRUNLENGTH"=34020, "IT8BITSPEREXTENDEDRUNLENGTH"=34021, "IT8COLORTABLE"=34022, "IT8IMAGECOLORINDICATOR"=34023, "IT8BKGCOLORINDICATOR"=34024, "IT8IMAGECOLORVALUE"=34025, "IT8BKGCOLORVALUE"=34026, "IT8PIXELINTENSITYRANGE"=34027, "IT8TRANSPARENCYINDICATOR"=34028, "IT8COLORCHARACTERIZATION"=34029, "IT8HCUSAGE"=34030, "IT8TRAPINDICATOR"=34031, "IT8CMYKEQUIVALENT"=34032, "FRAMECOUNT"=34232, "PHOTOSHOP"=34377, "EXIFIFD"=34665, "ICCPROFILE"=34675, "JBIGOPTIONS"=34750, "EXIF_EXPOSUREPROGRAM"=34850, "EXIF_SPECTRALSENSITIVITY"=34852, "GPSIFD"=34853, "EXIF_ISOSPEEDRATINGS"=34855, "EXIF_OECF"=34856, "FAXRECVPARAMS"=34908, "FAXSUBADDRESS"=34909, "FAXRECVTIME"=34910, "FAXDCS"=34911, "FEDEX_EDR"=34929, "EXIF_EXIFVERSION"=36864, "EXIF_DATETIMEORIGINAL"=36867, "EXIF_DATETIMEDIGITIZED"=36868, "EXIF_COMPONENTSCONFIGURATION"=37121, "EXIF_COMPRESSEDBITSPERPIXEL"=37122, "EXIF_SHUTTERSPEEDVALUE"=37377, "EXIF_APERTUREVALUE"=37378, "EXIF_BRIGHTNESSVALUE"=37379, "EXIF_EXPOSUREBIASVALUE"=37380, "EXIF_MAXAPERTUREVALUE"=37381, "EXIF_SUBJECTDISTANCE"=37382, "EXIF_METERINGMODE"=37383, "EXIF_LIGHTSOURCE"=37384, "EXIF_FLASH"=37385, "EXIF_FOCALLENGTH"=37386, "EXIF_SUBJECTAREA"=37396, "STONITS"=37439, "EXIF_MAKERNOTE"=37500, "EXIF_USERCOMMENT"=37510, "EXIF_SUBSECTIME"=37520, "EXIF_SUBSECTIMEORIGINAL"=37521, "EXIF_SUBSECTIMEDIGITIZED"=37522, "EXIF_FLASHPIXVERSION"=40960, "EXIF_COLORSPACE"=40961, "EXIF_PIXELXDIMENSION"=40962, "EXIF_PIXELYDIMENSION"=40963, "EXIF_RELATEDSOUNDFILE"=40964, "INTEROPERABILITYIFD"=40965, "EXIF_FLASHENERGY"=41483, "EXIF_SPATIALFREQUENCYRESPONSE"=41484, "EXIF_FOCALPLANEXRESOLUTION"=41486, "EXIF_FOCALPLANEYRESOLUTION"=41487, "EXIF_FOCALPLANERESOLUTIONUNIT"=41488, "EXIF_SUBJECTLOCATION"=41492, "EXIF_EXPOSUREINDEX"=41493, "EXIF_SENSINGMETHOD"=41495, "EXIF_FILESOURCE"=41728, "EXIF_SCENETYPE"=41729, "EXIF_CFAPATTERN"=41730, "EXIF_CUSTOMRENDERED"=41985, "EXIF_EXPOSUREMODE"=41986, "EXIF_WHITEBALANCE"=41987, "EXIF_DIGITALZOOMRATIO"=41988, "EXIF_FOCALLENGTHIN35MMFILM"=41989, "EXIF_SCENECAPTURETYPE"=41990, "EXIF_GAINCONTROL"=41991, "EXIF_CONTRAST"=41992, "EXIF_SATURATION"=41993, "EXIF_SHARPNESS"=41994, "EXIF_DEVICESETTINGDESCRIPTION"=41995, "EXIF_SUBJECTDISTANCERANGE"=41996, "EXIF_IMAGEUNIQUEID"=42016, "DNGVERSION"=50706, "DNGBACKWARDVERSION"=50707, "UNIQUECAMERAMODEL"=50708, "LOCALIZEDCAMERAMODEL"=50709, "CFAPLANECOLOR"=50710, "CFALAYOUT"=50711, "LINEARIZATIONTABLE"=50712, "BLACKLEVELREPEATDIM"=50713, "BLACKLEVEL"=50714, "BLACKLEVELDELTAH"=50715, "BLACKLEVELDELTAV"=50716, "WHITELEVEL"=50717, "DEFAULTSCALE"=50718, "DEFAULTCROPORIGIN"=50719, "DEFAULTCROPSIZE"=50720, "COLORMATRIX1"=50721, "COLORMATRIX2"=50722, "CAMERACALIBRATION1"=50723, "CAMERACALIBRATION2"=50724, "REDUCTIONMATRIX1"=50725, "REDUCTIONMATRIX2"=50726, "ANALOGBALANCE"=50727, "ASSHOTNEUTRAL"=50728, "ASSHOTWHITEXY"=50729, "BASELINEEXPOSURE"=50730, "BASELINENOISE"=50731, "BASELINESHARPNESS"=50732, "BAYERGREENSPLIT"=50733, "LINEARRESPONSELIMIT"=50734, "CAMERASERIALNUMBER"=50735, "LENSINFO"=50736, "CHROMABLURRADIUS"=50737, "ANTIALIASSTRENGTH"=50738, "SHADOWSCALE"=50739, "DNGPRIVATEDATA"=50740, "MAKERNOTESAFETY"=50741, "CALIBRATIONILLUMINANT1"=50778, "CALIBRATIONILLUMINANT2"=50779, "BESTQUALITYSCALE"=50780, "RAWDATAUNIQUEID"=50781, "ORIGINALRAWFILENAME"=50827, "ORIGINALRAWFILEDATA"=50828, "ACTIVEAREA"=50829, "MASKEDAREAS"=50830, "ASSHOTICCPROFILE"=50831, "ASSHOTPREPROFILEMATRIX"=50832, "CURRENTICCPROFILE"=50833, "CURRENTPREPROFILEMATRIX"=50834, "DCSHUESHIFTVALUES"=65535, "FAXMODE"=65536, "JPEGQUALITY"=65537, "JPEGCOLORMODE"=65538, "JPEGTABLESMODE"=65539, "FAXFILLFUNC"=65540, "PIXARLOGDATAFMT"=65549, "DCSIMAGERTYPE"=65550, "DCSINTERPMODE"=65551, "DCSBALANCEARRAY"=65552, "DCSCORRECTMATRIX"=65553, "DCSGAMMA"=65554, "DCSTOESHOULDERPTS"=65555, "DCSCALIBRATIONFD"=65556, "ZIPQUALITY"=65557, "PIXARLOGQUALITY"=65558, "DCSCLIPRECTANGLE"=65559, "SGILOGDATAFMT"=65560, "SGILOGENCODE"=65561] ("tag")
        w129 = 256 items=["IGNORE"=0, "SUBFILETYPE"=254, "OSUBFILETYPE"=255, "IMAGEWIDTH"=256, "IMAGELENGTH"=257, "BITSPERSAMPLE"=258, "COMPRESSION"=259, "PHOTOMETRIC"=262, "THRESHHOLDING"=263, "CELLWIDTH"=264, "CELLLENGTH"=265, "FILLORDER"=266, "DOCUMENTNAME"=269, "IMAGEDESCRIPTION"=270, "MAKE"=271, "MODEL"=272, "STRIPOFFSETS"=273, "ORIENTATION"=274, "SAMPLESPERPIXEL"=277, "ROWSPERSTRIP"=278, "STRIPBYTECOUNTS"=279, "MINSAMPLEVALUE"=280, "MAXSAMPLEVALUE"=281, "XRESOLUTION"=282, "YRESOLUTION"=283, "PLANARCONFIG"=284, "PAGENAME"=285, "XPOSITION"=286, "YPOSITION"=287, "FREEOFFSETS"=288, "FREEBYTECOUNTS"=289, "GRAYRESPONSEUNIT"=290, "GRAYRESPONSECURVE"=291, "GROUP3OPTIONS, T4OPTIONS"=292, "GROUP4OPTIONS, T6OPTIONS"=293, "RESOLUTIONUNIT"=296, "PAGENUMBER"=297, "COLORRESPONSEUNIT"=300, "TRANSFERFUNCTION"=301, "SOFTWARE"=305, "DATETIME"=306, "ARTIST"=315, "HOSTCOMPUTER"=316, "PREDICTOR"=317, "WHITEPOINT"=318, "PRIMARYCHROMATICITIES"=319, "COLORMAP"=320, "HALFTONEHINTS"=321, "TILEWIDTH"=322, "TILELENGTH"=323, "TILEOFFSETS"=324, "TILEBYTECOUNTS"=325, "BADFAXLINES"=326, "CLEANFAXDATA"=327, "CONSECUTIVEBADFAXLINES"=328, "SUBIFD"=330, "INKSET"=332, "INKNAMES"=333, "NUMBEROFINKS"=334, "DOTRANGE"=336, "TARGETPRINTER"=337, "EXTRASAMPLES"=338, "SAMPLEFORMAT"=339, "SMINSAMPLEVALUE"=340, "SMAXSAMPLEVALUE"=341, "CLIPPATH"=343, "XCLIPPATHUNITS"=344, "YCLIPPATHUNITS"=345, "INDEXED"=346, "JPEGTABLES"=347, "OPIPROXY"=351, "JPEGPROC"=512, "JPEGIFOFFSET"=513, "JPEGIFBYTECOUNT"=514, "JPEGRESTARTINTERVAL"=515, "JPEGLOSSLESSPREDICTORS"=517, "JPEGPOINTTRANSFORM"=518, "JPEGQTABLES"=519, "JPEGDCTABLES"=520, "JPEGACTABLES"=521, "YCBCRCOEFFICIENTS"=529, "YCBCRSUBSAMPLING"=530, "YCBCRPOSITIONING"=531, "REFERENCEBLACKWHITE"=532, "XMLPACKET"=700, "OPIIMAGEID"=32781, "REFPTS"=32953, "REGIONTACKPOINT"=32954, "REGIONWARPCORNERS"=32955, "REGIONAFFINE"=32956, "MATTEING"=32995, "DATATYPE"=32996, "IMAGEDEPTH"=32997, "TILEDEPTH"=32998, "PIXAR_IMAGEFULLWIDTH"=33300, "PIXAR_IMAGEFULLLENGTH"=33301, "PIXAR_TEXTUREFORMAT"=33302, "PIXAR_WRAPMODES"=33303, "PIXAR_FOVCOT"=33304, "PIXAR_MATRIX_WORLDTOSCREEN"=33305, "PIXAR_MATRIX_WORLDTOCAMERA"=33306, "WRITERSERIALNUMBER"=33405, "COPYRIGHT"=33432, "EXIF_EXPOSURETIME"=33434, "EXIF_FNUMBER"=33437, "RICHTIFFIPTC"=33723, "IT8SITE"=34016, "IT8COLORSEQUENCE"=34017, "IT8HEADER"=34018, "IT8RASTERPADDING"=34019, "IT8BITSPERRUNLENGTH"=34020, "IT8BITSPEREXTENDEDRUNLENGTH"=34021, "IT8COLORTABLE"=34022, "IT8IMAGECOLORINDICATOR"=34023, "IT8BKGCOLORINDICATOR"=34024, "IT8IMAGECOLORVALUE"=34025, "IT8BKGCOLORVALUE"=34026, "IT8PIXELINTENSITYRANGE"=34027, "IT8TRANSPARENCYINDICATOR"=34028, "IT8COLORCHARACTERIZATION"=34029, "IT8HCUSAGE"=34030, "IT8TRAPINDICATOR"=34031, "IT8CMYKEQUIVALENT"=34032, "FRAMECOUNT"=34232, "PHOTOSHOP"=34377, "EXIFIFD"=34665, "ICCPROFILE"=34675, "JBIGOPTIONS"=34750, "EXIF_EXPOSUREPROGRAM"=34850, "EXIF_SPECTRALSENSITIVITY"=34852, "GPSIFD"=34853, "EXIF_ISOSPEEDRATINGS"=34855, "EXIF_OECF"=34856, "FAXRECVPARAMS"=34908, "FAXSUBADDRESS"=34909, "FAXRECVTIME"=34910, "FAXDCS"=34911, "FEDEX_EDR"=34929, "EXIF_EXIFVERSION"=36864, "EXIF_DATETIMEORIGINAL"=36867, "EXIF_DATETIMEDIGITIZED"=36868, "EXIF_COMPONENTSCONFIGURATION"=37121, "EXIF_COMPRESSEDBITSPERPIXEL"=37122, "EXIF_SHUTTERSPEEDVALUE"=37377, "EXIF_APERTUREVALUE"=37378, "EXIF_BRIGHTNESSVALUE"=37379, "EXIF_EXPOSUREBIASVALUE"=37380, "EXIF_MAXAPERTUREVALUE"=37381, "EXIF_SUBJECTDISTANCE"=37382, "EXIF_METERINGMODE"=37383, "EXIF_LIGHTSOURCE"=37384, "EXIF_FLASH"=37385, "EXIF_FOCALLENGTH"=37386, "EXIF_SUBJECTAREA"=37396, "STONITS"=37439, "EXIF_MAKERNOTE"=37500, "EXIF_USERCOMMENT"=37510, "EXIF_SUBSECTIME"=37520, "EXIF_SUBSECTIMEORIGINAL"=37521, "EXIF_SUBSECTIMEDIGITIZED"=37522, "EXIF_FLASHPIXVERSION"=40960, "EXIF_COLORSPACE"=40961, "EXIF_PIXELXDIMENSION"=40962, "EXIF_PIXELYDIMENSION"=40963, "EXIF_RELATEDSOUNDFILE"=40964, "INTEROPERABILITYIFD"=40965, "EXIF_FLASHENERGY"=41483, "EXIF_SPATIALFREQUENCYRESPONSE"=41484, "EXIF_FOCALPLANEXRESOLUTION"=41486, "EXIF_FOCALPLANEYRESOLUTION"=41487, "EXIF_FOCALPLANERESOLUTIONUNIT"=41488, "EXIF_SUBJECTLOCATION"=41492, "EXIF_EXPOSUREINDEX"=41493, "EXIF_SENSINGMETHOD"=41495, "EXIF_FILESOURCE"=41728, "EXIF_SCENETYPE"=41729, "EXIF_CFAPATTERN"=41730, "EXIF_CUSTOMRENDERED"=41985, "EXIF_EXPOSUREMODE"=41986, "EXIF_WHITEBALANCE"=41987, "EXIF_DIGITALZOOMRATIO"=41988, "EXIF_FOCALLENGTHIN35MMFILM"=41989, "EXIF_SCENECAPTURETYPE"=41990, "EXIF_GAINCONTROL"=41991, "EXIF_CONTRAST"=41992, "EXIF_SATURATION"=41993, "EXIF_SHARPNESS"=41994, "EXIF_DEVICESETTINGDESCRIPTION"=41995, "EXIF_SUBJECTDISTANCERANGE"=41996, "EXIF_IMAGEUNIQUEID"=42016, "DNGVERSION"=50706, "DNGBACKWARDVERSION"=50707, "UNIQUECAMERAMODEL"=50708, "LOCALIZEDCAMERAMODEL"=50709, "CFAPLANECOLOR"=50710, "CFALAYOUT"=50711, "LINEARIZATIONTABLE"=50712, "BLACKLEVELREPEATDIM"=50713, "BLACKLEVEL"=50714, "BLACKLEVELDELTAH"=50715, "BLACKLEVELDELTAV"=50716, "WHITELEVEL"=50717, "DEFAULTSCALE"=50718, "DEFAULTCROPORIGIN"=50719, "DEFAULTCROPSIZE"=50720, "COLORMATRIX1"=50721, "COLORMATRIX2"=50722, "CAMERACALIBRATION1"=50723, "CAMERACALIBRATION2"=50724, "REDUCTIONMATRIX1"=50725, "REDUCTIONMATRIX2"=50726, "ANALOGBALANCE"=50727, "ASSHOTNEUTRAL"=50728, "ASSHOTWHITEXY"=50729, "BASELINEEXPOSURE"=50730, "BASELINENOISE"=50731, "BASELINESHARPNESS"=50732, "BAYERGREENSPLIT"=50733, "LINEARRESPONSELIMIT"=50734, "CAMERASERIALNUMBER"=50735, "LENSINFO"=50736, "CHROMABLURRADIUS"=50737, "ANTIALIASSTRENGTH"=50738, "SHADOWSCALE"=50739, "DNGPRIVATEDATA"=50740, "MAKERNOTESAFETY"=50741, "CALIBRATIONILLUMINANT1"=50778, "CALIBRATIONILLUMINANT2"=50779, "BESTQUALITYSCALE"=50780, "RAWDATAUNIQUEID"=50781, "ORIGINALRAWFILENAME"=50827, "ORIGINALRAWFILEDATA"=50828, "ACTIVEAREA"=50829, "MASKEDAREAS"=50830, "ASSHOTICCPROFILE"=50831, "ASSHOTPREPROFILEMATRIX"=50832, "CURRENTICCPROFILE"=50833, "CURRENTPREPROFILEMATRIX"=50834, "DCSHUESHIFTVALUES"=65535, "FAXMODE"=65536, "JPEGQUALITY"=65537, "JPEGCOLORMODE"=65538, "JPEGTABLESMODE"=65539, "FAXFILLFUNC"=65540, "PIXARLOGDATAFMT"=65549, "DCSIMAGERTYPE"=65550, "DCSINTERPMODE"=65551, "DCSBALANCEARRAY"=65552, "DCSCORRECTMATRIX"=65553, "DCSGAMMA"=65554, "DCSTOESHOULDERPTS"=65555, "DCSCALIBRATIONFD"=65556, "ZIPQUALITY"=65557, "PIXARLOGQUALITY"=65558, "DCSCLIPRECTANGLE"=65559, "SGILOGDATAFMT"=65560, "SGILOGENCODE"=65561] ("tag")
        # "channel count"
        # "channel count"
        # "Fillorder is different from sample format:\none is the byte order (most significant to least significant byte or the other way round,\nwhich corresponds to dos/windows-like and unix-like systems)\nand sample format is signed or unsigned integers or floating point,...\nIt is not set in your blobs.tif and not used anyways"
        # "corresponds to \"getTag_SampleFormat\" in libtiff2.lvlib\n(not used)"
        n4 = invoke class="Tiff" method="GetField"(reference=w101, "tag"=w103) -> (reference out=w100:refnum<k24>, "GetField"=w99:refnum<k24>[])  [unwired: 2 in, 2 out]
        n5 = Index Array(array=w99) -> (element=w98:refnum<k24>)  [unwired: 1 in]
        n6 = property class="FieldValue"(reference=w98) -> ("Value"=w97:refnum<k24>)  [unwired: 1 in, 2 out]
        n7 = invoke class="Tiff" method="GetField"(reference=w100, error in=w102, "tag"=w129) -> (reference out=w136:refnum<k24>, error out=w131:errorcluster, "GetField"=w128:refnum<k24>[])  [unwired: 1 in, 1 out]
        n8 = for {
          tunnel: w128 -> [w205] mode=indexing
          tunnel: [w199] -> w127 mode=indexing
          n9 = property class="FieldValue"(reference=w205) -> (error out=w203:errorcluster, "Value"=w204:refnum<k24>)  [unwired: 1 in, 1 out]
          n10 = call <vilib>:".NET Object to Variant.vi"("error in (no error)"=w203, ".NET object"=w204) -> ("error out"=w202:errorcluster, "variant"=w201:variant)
          n11 = Variant To Data(error in=w202, type=0, Variant=w201) -> (data=w199:i32)  [unwired: 1 out]
        }
        n12 = call <vilib>:".NET Object to Variant.vi"(".NET object"=w97) -> ("error out"=w71:errorcluster, "variant"=w96:variant)  [unwired: 1 in]
        n13 = Variant To Data(error in=w71, type=variant[] [], Variant=w96) -> (data=w94:variant[])  [unwired: 1 out]
        n14 = for {
          tunnel: w94 -> [w169] mode=indexing
          tunnel: [w166] -> w72 mode=concatenating
          n15 = Variant To Data(type=u8 0, Variant=w169) -> (data=w168:u8)  [unwired: 1 in, 1 out]
          n16 = Type Cast(type="", x=w168) -> (*(type *) &x=w166:string)
        }
        "Subject" <- w72
        n17 = invoke class="Tiff" method="GetField"(reference=w136, error in=w131, "tag"=w135) -> (reference out=w134:refnum<k24>, error out=w132:errorcluster, "GetField"=w124:refnum<k24>[])  [unwired: 1 in, 1 out]
        n18 = for {
          tunnel: [w193] -> w125 mode=indexing
          tunnel: w124 -> [w192] mode=indexing
          n19 = property class="FieldValue"(reference=w192) -> (error out=w197:errorcluster, "Value"=w198:refnum<k24>)  [unwired: 1 in, 1 out]
          n20 = call <vilib>:".NET Object to Variant.vi"("error in (no error)"=w197, ".NET object"=w198) -> ("error out"=w196:errorcluster, "variant"=w195:variant)
          n21 = Variant To Data(error in=w196, type=0, Variant=w195) -> (data=w193:i32)  [unwired: 1 out]
        }
        n22 = Index Array(array=w127) -> (element=w126:i32)  [unwired: 1 in]
        n23 = Index Array(array=w125) -> (element=w123:i32)  [unwired: 1 in]
        n24 = invoke class="Tiff" method="GetField"(reference=w134, error in=w132, "tag"=w130) -> (reference out=w116:refnum<k24>, error out=w133:errorcluster, "GetField"=w121:refnum<k24>[])  [unwired: 1 in, 1 out]
        n25 = for {
          tunnel: [w186] -> w122 mode=indexing
          tunnel: w121 -> [w185] mode=indexing
          n26 = property class="FieldValue"(reference=w185) -> (error out=w190:errorcluster, "Value"=w191:refnum<k24>)  [unwired: 1 in, 1 out]
          n27 = call <vilib>:".NET Object to Variant.vi"("error in (no error)"=w190, ".NET object"=w191) -> ("error out"=w189:errorcluster, "variant"=w188:variant)
          n28 = Variant To Data(error in=w189, type=0, Variant=w188) -> (data=w186:i32)  [unwired: 1 out]
        }
        n29 = Index Array(array=w122) -> (element=w120:i32)  [unwired: 1 in]
        n30 = call <vilib>:"Parse JSON.vi"("JSON String"=w72) -> ("error out"=w78:errorcluster, "JSON Tree"=w79:variant)  [unwired: 7 in, 2 out]
        n31 = call-poly <vilib>:"Get Object Parameter.vi"("error in (no error)"=w78, "Parameter Name"="channels", "JSON Tree In (JSON Object)"=w79) -> ("error out"=w80:errorcluster, "JSON Object"=w85:variant)  [unwired: 5 in, 2 out]
        n32 = call-poly <vilib>:"Get Object Parameter.vi"("error in (no error)"=w78, "Parameter Name"="materials", "JSON Tree In (JSON Object)"=w79) -> ("error out"=w77:errorcluster, "JSON Object"=w86:variant)  [unwired: 5 in, 2 out]
        n33 = call <vilib>:"JSON Array Size.vi"("error in (no error)"=w80, "JSON Tree In (JSON Array)"=w85) -> ("error out"=w81:errorcluster, "Array Size"=w84:i32, "JSON Tree Passthrough (JSON Array)"=w83:variant)  [unwired: 7 in]
        n34 = call-poly <vilib>:"Get Object Parameter.vi"("error in (no error)"=w77, "Parameter Name"="names", "JSON Tree In (JSON Object)"=w86) -> ("error out"=w76:errorcluster, "JSON Object"=w90:variant)  [unwired: 5 in, 2 out]
        n35 = for {
          N: w84 -> [_]
          tunnel: w83 -> [w157]
          tunnel: [w153] -> w69 mode=indexing
          tunnel: [w144] -> w74 mode=indexing
          tunnel: w81 -> [w143]
          i -> [w149]
          n36 = call <vilib>:"Node Type.vi"("error in (no error)"=w143, "JSON Tree In"=w157) -> ("error out"=w148:errorcluster, "Value"=w156:variant)  [unwired: 5 in, 3 out]
          n37 = call <vilib>:"JSON Array Size.vi"("error in (no error)"=w148, "JSON Tree In (JSON Array)"=w156) -> ("error out"=w147:errorcluster, "JSON Tree Passthrough (JSON Array)"=w155:variant)  [unwired: 7 in, 1 out]
          n38 = call-poly <vilib>:"Get Array Value at Index.vi"("error in (no error)"=w147, "Index"=w149, "JSON Tree In (JSON Array)"=w155) -> ("error out"=w146:errorcluster, "JSON Array"=w154:variant)  [unwired: 5 in, 2 out]
          n39 = call-poly <vilib>:"Get Object Parameter.vi"("error in (no error)"=w146, "Parameter Name"="targetMaterial", "JSON Tree In (JSON Object)"=w154) -> ("error out"=w145:errorcluster, "JSON Object"=w151:variant)  [unwired: 5 in, 2 out]
          n40 = Variant To Data(error in=w145, type="", Variant=w151) -> (data=w153:string, error out=w144:errorcluster)
        }
        n41 = call <vilib>:"JSON Array Size.vi"("error in (no error)"=w76, "JSON Tree In (JSON Array)"=w90) -> ("error out"=w82:errorcluster, "Array Size"=w87:i32, "JSON Tree Passthrough (JSON Array)"=w89:variant)  [unwired: 7 in]
        n42 = call <vilib>:"Node Type.vi"("error in (no error)"=w82, "JSON Tree In"=w89) -> ("Value"=w88:variant)  [unwired: 5 in, 4 out]
        n43 = for {
          N: w87 -> [_]
          shift-right: [w164] -> _
          shift-left: w88 -> [w165]
          tunnel: [w160] -> w68 mode=indexing
          tunnel: [w158] -> w75 mode=indexing
          i -> [w163]
          n44 = call-poly <vilib>:"Get Array Value at Index.vi"("Index"=w163, "JSON Tree In (JSON Array)"=w165) -> ("error out"=w159:errorcluster, "JSON Array"=w162:variant, "JSON Tree Out Passthrough"=w164:variant)  [unwired: 6 in, 1 out]
          n45 = Variant To Data(error in=w159, type="", Variant=w162) -> (data=w160:string, error out=w158:errorcluster)
        }
        n46 = case shown="8" w120 {
          selector: w120 -> [_ w248 _ w294 _ w366]
          tunnel: [w221 w251 TRUE w305 w345 w369] -> w142
          tunnel: w126 -> [w206 w250 _ w297 _ w368]
          tunnel: w123 -> [w207 w249 _ w298 w337 w367]
          tunnel: [_ _ _ w291 w335 w365] -> w114
          tunnel: [w228 _ _ _ _ _] -> w137
          tunnel: [_ w247 _ _ _ _] -> w140
          tunnel: w116 -> [w225 w246 w284 w308 w348 w364]
          tunnel: w133 -> [w224 w245 w283 w307 w347 w363]
          tunnel: [w219 w245 w283 w303 w343 w363] -> w138
          tunnel: [w218 w246 w284 w290 w340 w364] -> w139
          tunnel: [_ _ _ w286 _ _] -> _
          tunnel: [_ _ _ _ w334 _] -> w108
          tunnel: [_ _ _ _ w333 _] -> w107
          tunnel: [_ _ _ _ w332 _] -> w106
          tunnel: [_ _ _ _ w331 _] -> w105
          tunnel: [_ _ _ _ w330 _] -> w104
          tunnel: [_ _ _ _ w329 _] -> w70
          frame 16 {
            w215 = 2  # Bytes  per pxl
            w226 = u8 0  # Element (U8)
            # "Grayscale U16"
            # "Create buffer"
            n47 = invoke class="Tiff" method="NumberOfStrips"(reference=w225, error in=w224) -> (reference out=w223:refnum<k24>, error out=w229:errorcluster, "NumberOfStrips"=w212:i32)  [unwired: 1 in]
            n48 = Compound Arithmetic op=MULTIPLY(w215, w207, w206) -> (w216:i32)
            n49 = Initialize Array(w226, w216) -> (w227:u8[])
            n50 = for {
              N: w212 -> [_]
              shift-right: [w231] -> w211
              shift-left: w227 -> [w234]
              tunnel: w223 -> [w244]
              tunnel: [w237] -> w222
              shift-right: [w236] -> w220
              shift-left: w229 -> [w239]
              shift-right: [w233] -> w213
              shift-left: 0 ("ReadEncodedStrip") -> [w230]
              i -> [w243]
              stop <- w235 stop-if-true
              # "Count bytes"
              n51 = invoke class="Tiff" method="RawStripSize"(reference=w244, error in=w239, "strip"=w243) -> (reference out=w240:refnum<k24>, error out=w238:errorcluster, "RawStripSize"=w242:i64)  [unwired: 1 in, 1 out]
              n52 = To Long Integer(number=w242) -> (32bit integer=w241:i32)
              n53 = invoke class="Tiff" method="ReadRawStrip"(reference=w240, error in=w238, "strip"=w243, "buffer"=w234, "offset"=w230, "count"=w241) -> (reference out=w237:refnum<k24>, error out=w236:errorcluster, "ReadRawStrip"=w232:i32, "buffer"=w231:u8[])  [unwired: 1 in, 3 out]
              n54 = Unbundle(w236) -> ("status"=w235:bool)  [unwired: 2 out]
              n55 = Add(x=w232, y=w230) -> (x+y=w233:i32)
            }
            "Number Bytes read" <- w213
            n56 = invoke class="Tiff" method="ReadDirectory"(reference=w222, error in=w220) -> (reference out=w218:refnum<k24>, error out=w219:errorcluster, "ReadDirectory"=w217:bool)  [unwired: 1 in]
            n57 = Decimate 1D Array(w211) -> (w208:u8[], w209:u8[])
            n58 = Join Numbers(hi=w209, lo=w208) -> ((hi.lo)=w210:u16[])
            n59 = Not(x=w217) -> (.not. x?=w221:bool)
            n60 = Reshape Array(w210, w207, w206) -> (w228:u16[][])
          }
          frame 32 {
            n61 = disable-structure shown="Disabled" {
              disable-tunnel: [w267 TRUE] -> w251
              disable-tunnel: w250 -> [w262 _]
              disable-tunnel: w249 -> [w261 _]
              disable-tunnel: w248 -> [w255 _]
              disable-tunnel: [w252 _] -> w247
              frame Disabled {
                w256 = sgl 0.0 ("element")
                # "Grayscale U32"
                # "Create buffer"
                # "number of strips"
                # "read directory"
                n62 = dll-call lib="BitMiracle.LibTiff.NET.dll" fn="TIFFNumberOfStrips"() -> (error out=w259:errorcluster, "return type"=w264:u32, "handle"=w265:i32)  [unwired: 4 in, 1 out]
                n63 = Divide(x=w255, y=u32 8) -> (x/y=w253:dbl)
                n64 = Initialize Array(w256, w256) -> (w257:sgl[])
                n65 = for {
                  N: w264 -> [_]
                  tunnel: [w281] -> w263
                  tunnel: w265 -> [w279]
                  tunnel: [w274] -> w260 mode=indexing
                  tunnel: w259 -> [w277]
                  tunnel: [w280] -> w258
                  shift-right: [w274] -> _
                  shift-left: w257 -> [w273]
                  tunnel: w253 -> [w270]
                  tunnel: [w268] -> _ mode=indexing
                  i -> [w278]
                  # "read raw strip size"
                  # "read encoded strip"
                  n66 = dll-call lib="BitMiracle.LibTiff.NET.dll" fn="TIFFRawStripSize"(error in=w277, "handle"=w279, "strip"=w278) -> (error out=w276:errorcluster, "return type"=w271:u32, "handle"=w275:i32)  [unwired: 3 in, 1 out]
                  n67 = Divide(x=w271, y=w270) -> (x/y=w269:dbl)
                  n68 = Reshape Array(w273, w269) -> (w272:sgl[])
                  n69 = dll-call lib="BitMiracle.LibTiff.NET.dll" fn="TIFFReadEncodedStrip"(error in=w276, "Handle"=w275, "strip"=w278, "buffer"=w272, "length"=w271) -> (error out=w280:errorcluster, "return type"=w268:u32, "Handle"=w281:i32, "buffer"=w274:sgl[])  [unwired: 4 in, 1 out]
                }
                n70 = dll-call lib="BitMiracle.LibTiff.NET.dll" fn="TIFFReadDirectory"(error in=w258, "handle"=w263) -> ("return type"=w266:i32)  [unwired: 3 in, 2 out]
                n71 = Reshape Array(w260, w261, w262) -> (w252:sgl[][])
                n72 = Equal To 0?(x=w266) -> (x = 0?=w267:bool)
              }
              frame Enabled {
              }
            }
          }
          frame 0, Default {
            (unwired) errorcluster {"status"=TRUE, "code"=5000, "source"="Unsupported TIFF format"} ("error out")
          }
          frame 82 {
            w296 = u8 0 ("element")
            # "Grayscale U8"
            # "Create buffer"
            n73 = invoke class="Tiff" method="NumberOfStrips"(reference=w308, error in=w307) -> (reference out=w287:refnum<k24>, error out=w309:errorcluster, "NumberOfStrips"=w299:i32)  [unwired: 1 in]
            n74 = Divide(x=w294, y=u32 8) -> (x/y=w292:dbl)
            n75 = Initialize Array(w296, w296) -> (w295:u8[])
            n76 = for {
              N: w299 -> [_]
              shift-right: [w310] -> w288
              shift-left: w295 -> [w314]
              tunnel: w287 -> [w328]
              tunnel: [w322] -> w306
              shift-right: [w321] -> w304
              shift-left: w309 -> [w324]
              shift-right: [w319] -> w300
              shift-left: 0 ("ReadEncodedStrip") -> [w312]
              tunnel: w292 -> [w316]
              tunnel: [w310] -> w286 mode=indexing
              i -> [w327]
              stop <- w320 stop-if-true
              # "Count bytes"
              n77 = invoke class="Tiff" method="RawStripSize"(reference=w328, error in=w324, "strip"=w327) -> (reference out=w325:refnum<k24>, error out=w323:errorcluster, "RawStripSize"=w317:i64)  [unwired: 1 in, 1 out]
              n78 = Divide(x=w317, y=w316) -> (x/y=w315:dbl)
              n79 = To Long Integer(number=w317) -> (32bit integer=w326:i32)
              n80 = Reshape Array(w314, w315) -> (w313:u8[])
              n81 = invoke class="Tiff" method="ReadRawStrip"(reference=w325, error in=w323, "strip"=w327, "buffer"=w313, "offset"=0, "count"=w326) -> (reference out=w322:refnum<k24>, error out=w321:errorcluster, "ReadRawStrip"=w318:i32, "buffer"=w310:u8[])  [unwired: 1 in, 3 out]
              n82 = Unbundle(w321) -> ("status"=w320:bool)  [unwired: 2 out]
              n83 = Add(x=w318, y=w312) -> (x+y=w319:i32)
            }
            "Number Bytes read 2" <- w300
            "Array" <- w288
            "buffer" <- w286
            n84 = invoke class="Tiff" method="ReadDirectory"(reference=w306, error in=w304) -> (reference out=w290:refnum<k24>, error out=w303:errorcluster, "ReadDirectory"=w302:bool)  [unwired: 1 in]
            n85 = Not(x=w302) -> (.not. x?=w305:bool)
            n86 = invoke class="Tiff" method="NumberOfTiles"(reference=w290) -> ("NumberOfTiles"=→"NumberOfTiles":i32)  [unwired: 2 in, 2 out]
            n87 = Reshape Array(w288, w298, w297) -> (w291:u8[][])
          }
          frame 8 {
            # "Count bytes"
            # "Create buffer"
            n88 = invoke class="Tiff" method="ScanlineSize"(reference=w348, error in=w347) -> (reference out=w339:refnum<k24>, error out=w349:errorcluster, "ScanlineSize"=w336:i32)  [unwired: 1 in]
            "ScanLineSize" <- w336
            n89 = Initialize Array(u8 0 ("element"), w336) -> (w338:u8[])
            n90 = for {
              N: w337 -> [_]
              tunnel: w338 -> [w358]
              shift-right: [w361] -> w344
              shift-left: w349 -> [w359]
              shift-right: [w362] -> w346
              shift-left: w339 -> [w360]
              tunnel: [w356] -> w329 mode=indexing
              tunnel: [w355] -> w334 mode=indexing
              tunnel: [w354] -> w333 mode=indexing
              tunnel: [w353] -> w332 mode=indexing
              tunnel: [w352] -> w331 mode=indexing
              tunnel: [w351] -> w330 mode=indexing
              tunnel: [w350] -> w335 mode=indexing
              i -> [w357]
              (unwired) i16 0 ("plane")
              # "Grayscale U8"
              n91 = invoke class="Tiff" method="ReadScanline"(reference=w360, error in=w359, "buffer"=w358, "row"=w357) -> (reference out=w362:refnum<k24>, error out=w361:errorcluster, "buffer"=w356:u8[])  [unwired: 1 in, 2 out]
              n92 = Decimate 1D Array(w356) -> (w355:u8[], w354:u8[], w353:u8[], w352:u8[], w351:u8[], w350:u8[])
            }
            n93 = invoke class="Tiff" method="ReadDirectory"(reference=w346, error in=w344) -> (reference out=w340:refnum<k24>, error out=w343:errorcluster, "ReadDirectory"=w342:bool)  [unwired: 1 in]
            n94 = Not(x=w342) -> (.not. x?=w345:bool)
            "Numeric" <- w337
          }
          frame 81 {
            n95 = disable-structure shown="Enabled" {
              disable-tunnel: [w385 TRUE] -> w369
              disable-tunnel: w368 -> [w380 _]
              disable-tunnel: w367 -> [w379 _]
              disable-tunnel: w366 -> [w373 _]
              disable-tunnel: [w370 _] -> w365
              frame Disabled {
                w374 = u8 0 ("element")
                # "Grayscale U8"
                # "Create buffer"
                # "number of strips"
                # "read directory"
                n96 = dll-call lib="BitMiracle.LibTiff.NET.dll" fn="TIFFNumberOfStrips"() -> (error out=w377:errorcluster, "return type"=w382:u32, "handle"=w383:i32)  [unwired: 4 in, 1 out]
                n97 = Divide(x=w373, y=u32 8) -> (x/y=w371:dbl)
                n98 = Initialize Array(w374, w374) -> (w375:u8[])
                n99 = for {
                  N: w382 -> [_]
                  tunnel: [w399] -> w381
                  tunnel: w383 -> [w397]
                  tunnel: [w392] -> w378 mode=indexing
                  tunnel: w377 -> [w395]
                  tunnel: [w398] -> w376
                  shift-right: [w392] -> _
                  shift-left: w375 -> [w391]
                  tunnel: w371 -> [w388]
                  tunnel: [w386] -> _ mode=indexing
                  i -> [w396]
                  # "read raw strip size"
                  # "read raw strip"
                  n100 = dll-call lib="BitMiracle.LibTiff.NET.dll" fn="TIFFRawStripSize"(error in=w395, "handle"=w397, "strip"=w396) -> (error out=w394:errorcluster, "return type"=w389:u32, "handle"=w393:i32)  [unwired: 3 in, 1 out]
                  n101 = Divide(x=w389, y=w388) -> (x/y=w387:dbl)
                  n102 = Reshape Array(w391, w387) -> (w390:u8[])
                  n103 = dll-call lib="BitMiracle.LibTiff.NET.dll" fn="TIFFReadRawStrip"(error in=w394, "Handle"=w393, "strip"=w396, "buffer"=w390, "length"=w389) -> (error out=w398:errorcluster, "return type"=w386:u32, "Handle"=w399:i32, "buffer"=w392:u8[])  [unwired: 4 in, 1 out]
                }
                n104 = dll-call lib="BitMiracle.LibTiff.NET.dll" fn="TIFFReadDirectory"(error in=w376, "handle"=w381) -> ("return type"=w384:i32)  [unwired: 3 in, 2 out]
                n105 = Reshape Array(w378, w379, w380) -> (w370:u8[][])
                n106 = Equal To 0?(x=w384) -> (x = 0?=w385:bool)
              }
              frame Enabled {
              }
            }
          }
        }
        n107 = invoke class="Tiff" method="GetField"(reference=w116, "tag"=w119) -> (reference out=w112:refnum<k24>, "GetField"=w117:refnum<k24>[])  [unwired: 2 in, 2 out]
        n108 = Merge Errors(w74, w75) -> (→"error out 2":errorcluster)
        n109 = invoke class="Tiff" method="GetField"(reference=w112, "tag"=w113) -> ("GetField"=w109:refnum<k24>[])  [unwired: 2 in, 3 out]
        n110 = for {
          tunnel: [w179] -> w118 mode=indexing
          tunnel: w117 -> [w178] mode=indexing
          n111 = property class="FieldValue"(reference=w178) -> (error out=w183:errorcluster, "Value"=w184:refnum<k24>)  [unwired: 1 in, 1 out]
          n112 = call <vilib>:".NET Object to Variant.vi"("error in (no error)"=w183, ".NET object"=w184) -> ("error out"=w182:errorcluster, "variant"=w181:variant)
          n113 = Variant To Data(error in=w182, type=0, Variant=w181) -> (data=w179:i32)  [unwired: 1 out]
        }
        n114 = for {
          tunnel: [w172] -> w110 mode=indexing
          tunnel: w109 -> [w171] mode=indexing
          n115 = property class="FieldValue"(reference=w171) -> (error out=w176:errorcluster, "Value"=w177:refnum<k24>)  [unwired: 1 in, 1 out]
          n116 = call <vilib>:".NET Object to Variant.vi"("error in (no error)"=w176, ".NET object"=w177) -> ("error out"=w175:errorcluster, "variant"=w174:variant)
          n117 = Variant To Data(error in=w175, type=0, Variant=w174) -> (data=w172:i32)  [unwired: 1 out]
        }
        n118 = Index Array(array=w118) -> (element=→"element":i32)  [unwired: 1 in]
        n119 = Index Array(array=w110) -> (element=→"element 2":i32)  [unwired: 1 in]
      }
      n120 = invoke class="Tiff" method="Close"(reference=w61, error in=w60) -> (error out=w59:errorcluster)  [unwired: 1 in, 2 out]
      n121 = Increment(x=w66) -> (x+1=w65:i32)
    }
    frame Error {
    }
  }
  "number of frames" <- w49
  "error out" <- w48
  "Grayscale (SGL) Image Data" <- w47
  "Grayscale (U16) Image Data" <- w44
  "unsigned 8bit integer" <- w37
  "ImageBufferMain" <- w3
  "ChannelTargetMaterials" <- w2
  "MaterialNames" <- w1
  n122 = disable-structure shown="Disabled" {
    frame Disabled {
    }
    frame Enabled {
    }
  }
  n123 = Bundle By Name(cluster=T1 {"ImageBufferMain"=[], "ChannelTargetMaterials"=[], "MaterialNames"=[]} ("ImageData"), "ImageBufferMain"=w3, "ChannelTargetMaterials"=w2, "MaterialNames"=w1) -> (→"ImageData":T1)
  n124 = call "IMAQ Create"("Image Name"="1", "Image Type"=w40) -> ("New Image"=w39:T2, "error out"=w22:errorcluster)  [unwired: 3 in]
  n125 = call "IMAQ Create"("Image Name"="2", "Image Type"=w36) -> ("New Image"=w25:T2, "error out"=w23:errorcluster)  [unwired: 3 in]
  n126 = call "IMAQ Create"("Image Name"="3", "Image Type"=w33) -> ("New Image"=w11:T2, "error out"=w10:errorcluster)  [unwired: 3 in]
  n127 = call "IMAQ Create"("Image Name"="4", "Image Type"=w29) -> ("New Image"=w18:T2, "error out"=w19:errorcluster)  [unwired: 3 in]
  n128 = call "IMAQ Create"("Image Name"="5", "Image Type"=w32) -> ("New Image"=w15:T2, "error out"=w16:errorcluster)  [unwired: 3 in]
  n129 = call "IMAQ Create"("Image Name"="6", "Image Type"=w27) -> ("New Image"=w12:T2, "error out"=w13:errorcluster)  [unwired: 3 in]
  n130 = call "IMAQ ArrayToImage"("error in (no error)"=w13, "Image Pixels (U8)"=w6, "Image"=w12) -> ("Image Out"=→"0 6":T2)  [unwired: 7 in, 1 out]
  n131 = call "IMAQ ArrayToImage"("error in (no error)"=w19, "Image Pixels (U8)"=w8, "Image"=w18) -> ("Image Out"=→"0 4":T2)  [unwired: 7 in, 1 out]
  n132 = call "IMAQ ArrayToImage"("error in (no error)"=w16, "Image Pixels (U8)"=w7, "Image"=w15) -> ("Image Out"=→"0 5":T2)  [unwired: 7 in, 1 out]
  n133 = call "IMAQ ArrayToImage"("error in (no error)"=w23, "Image Pixels (U8)"=w24, "Image"=w25) -> ("Image Out"=→"0 2":T2)  [unwired: 7 in, 1 out]
  n134 = call "IMAQ ArrayToImage"("error in (no error)"=w10, "Image Pixels (U8)"=w9, "Image"=w11) -> ("Image Out"=→"0 3":T2)  [unwired: 7 in, 1 out]
  n135 = call "IMAQ ArrayToImage"("error in (no error)"=w22, "Image Pixels (U8)"=w37, "Image"=w39) -> ("Image Out"=→"0":T2)  [unwired: 7 in, 1 out]
